vi "Transconductance state machine.vi"() -> ()   [LabVIEW 2016, in "Tranconductance SM.lvclass"]
uses:
  Tranconductance SM.lvclass
  <userlib>/LevyLab/Levylab Instruments/SMOs/Configuration/Configuration.lvclass
  <vilib>/Utility/sysdir.llb/System Directory Type.ctl
  Typedefs/Blob File--Cluster.ctl
  <userlib>/LevyLab/XY Utilities/Typedefs/Interpolation Configuration--cluster.ctl
  <userlib>/LevyLab/XY Utilities/subVIs/Remove Outliers (multiple).vi
  <userlib>/LevyLab/XY Utilities/subVIs/Zero Phase Lowpass Filter (multiple).vi
  <userlib>/LevyLab/XY Utilities/subVIs/Multiply float (multiple).vi
  <userlib>/LevyLab/XY Utilities/subVIs/Subtract float (multiple).vi
  <userlib>/LevyLab/XY Utilities/subVIs/Derivative (multiple).vi
  <userlib>/LevyLab/XY Utilities/subVIs/Interpolate (single).vi
  <vilib>/regexp/Match Regular Expression.xnode
  <vilib>/Analysis/NI_AAL_SigProc.lvlib
  <userlib>/LevyLab/Graph Utilities/graph_utilities.lvclass
  <userlib>/LevyLab/LV to ITX/Data.ITX/Data.ITX.lvclass
  <vilib>/Analysis/NI_AALPro.lvlib
  <userlib>/LevyLab/XY Utilities/xy_utilities.lvlib
  <userlib>/LevyLab/XY Utilities/subVIs/Shift Zero (single).vi
  <userlib>/LevyLab/LV to ITX/Data.TDMS/Data.TDMS.lvclass
  <userlib>/LevyLab/XY Utilities/subVIs/Resample (single).vi
  <userlib>/LevyLab/XY Utilities/subVIs/Subset (single).vi
panel:
  out "Current State":string
  in  "Clear Graphs & Stop":bool=TRUE
  in  "line cut":enum16{"Conductance", "Transconductance"}(ring)
  in  "Tab Control 2":T1(tab)
  out "Vertical Line Cut":cluster{"N1 (B field)":dbl[], dbl[]}[](graph)
  out "B field (T)":dbl=5.33284074074074
  out "vertical line cut \ncursor index":i32
  out "Horizontal Line Cut":cluster{"N1 (B field)":dbl[], dbl[]}[](graph)
  out "Vsg (V)":dbl=0.0006378350000000002 format="%#_6p"
  out "horizontal line cut\ncursor index":i32
  in  "Refresh":bool
  in  "Tab Control":T2(tab)
  in  "Load Notes":bool
  in  "B":u16(ring) items=["OFF", "Magnet Field", "Temperature", "Magnet", "Time", "Vsg", "X1", "Y1", "X2", "Y2", "X3", "Y3", "X4", "Y4", "X5", "Y5", "X6", "Y6", "X7", "Y7", "X8", "Y8"]
  in  "Vsg":u16(ring) items=["OFF", "Magnet Field", "Temperature", "Magnet", "Time", "Vsg", "X1", "Y1", "X2", "Y2", "X3", "Y3", "X4", "Y4", "X5", "Y5", "X6", "Y6", "X7", "Y7", "X8", "Y8"]
  in  "CURRENT":u16(ring) items=["OFF", "Magnet Field", "Temperature", "Magnet", "Time", "Vsg", "X1", "Y1", "X2", "Y2", "X3", "Y3", "X4", "Y4", "X5", "Y5", "X6", "Y6", "X7", "Y7", "X8", "Y8"]
  in  "V2":u16(ring) items=["OFF", "Magnet Field", "Temperature", "Magnet", "Time", "Vsg", "X1", "Y1", "X2", "Y2", "X3", "Y3", "X4", "Y4", "X5", "Y5", "X6", "Y6", "X7", "Y7", "X8", "Y8"]
  in  "Read TDMS Data":bool=TRUE
  in  "TDMS Path":path=path "G:/My Drive/ansom/Data/MNK/SA03018H.20170509/6 - sweep B, Vsg"
  in  "Load Wavenames":bool
  in  "V1":u16(ring) items=["OFF", "Magnet Field", "Temperature", "Magnet", "Time", "Vsg", "X1", "Y1", "X2", "Y2", "X3", "Y3", "X4", "Y4", "X5", "Y5", "X6", "Y6", "X7", "Y7", "X8", "Y8"]
  in  "Blob File Path":path=path "P:/users1/kirkendall/data/superlattice blob files/SA03018F.20171127_17B - sweep B, Vsg lockin, superlattice_original_6,8-4.blob"
  in  "Read Blob Data":bool
  in  "B field in T?":bool=TRUE
  in  "Indices":T3={"N1 (x axis)"=3, "N2"=19, "N3"=4, "N4"=5, "V1"=14, "V2"=4, "V3"=10, "V4"=13, "CURRENT"=6, "Vsg"=1}
  in  "ITX File or Folder Path":path=path "G:/My Drive/ansom/Data/MNK/SA03018H.20170509/6 - sweep B, Vsg"
  in  "File offset":i32
  in  "File length":i32=1000
  in  "single ended?":bool=TRUE
  in  "Read ITX Data":bool=TRUE
  out "Conductance vs Vsg":cluster{"N1 (B field)":dbl[], dbl[]}[](graph)
  out "Notes":string="IGOR\nX// Date: 2/8/2017 10:35 PM\nX// B=18T --> 0T, 0.05 T/min\nX// large axis: 157 -- 177, 10 deg steps\nX// small axis: 167\nX// sweep Vsg: 50mV to 170mV, 250uV steps\nX// Vbg=0.3V\nX// T<50mK\nX// \nX// lockin settings: \nX// tc=0.3s\nX// order=4\nX// prefilters OFF\nX// \nX// 0: 1, voltage\nX// 1: 2, current, 100uV AC 240uV DC, 13 Hz\nX// 2: 3, voltage\nX// 3: 4, voltage\nX// 4: 5, current\nX// 5: 7, voltage\nX//  \nX// KH gain=100x, shunt resistor=50kOhm\nX// \nX// axis1=157.013000\nX// axis2=166.999000\n\n\n\n\n\n\n\n\n\n\n\n\n\n\n\n\n\n\n\n\n\n\n\n\n\n\n\n\n\n\n\n\n\n\n\n\n\n\n\n\n\n\nX \nX Display/R 'time.SA02836H.20170110.000242'\nX AppendToGraph 'Vsg.SA02836H.20170110.000242'\nX AppendToGraph 'T.SA02836H.20170110.000242'\nX AppendToGraph 'B.SA02836H.20170110.000242'\nX AppendToGraph 'X0.SA02836H.20170110.000242'\nX AppendToGraph 'Y0.SA02836H.20170110.000242'\nX AppendToGraph 'X1.SA02836H.20170110.000242'\nX AppendToGraph 'Y1.SA02836H.20170110.000242'\nX AppendToGraph 'X2.SA02836H.20170110.000242'\nX AppendToGraph 'Y2.SA02836H.20170110.000242'\nX AppendToGraph 'X3.SA02836H.20170110.000242'\nX AppendToGraph 'Y3.SA02836H.20170110.000242'\nX AppendToGraph 'X4.SA02836H.20170110.000242'\nX AppendToGraph 'Y4.SA02836H.20170110.000242'\nX AppendToGraph 'X5.SA02836H.20170110.000242'\nX AppendToGraph 'Y5.SA02836H.20170110.000242'\nX AppendToGraph 'B_rate.SA02836H.20170110.000242'\nX AppendToGraph 'R4t(e2/h).SA02836H.20170110.000242'\nX AppendToGraph 'axis1.SA02836H.20170110.000242'\nX AppendToGraph 'axis2.SA02836H.20170110.000242'\nX Label bottom \"x label\"\nX Label left \"y label\"\nX ModifyGraph rgb('time.SA02836H.20170110.000242')=(65280,0,0)\nX ModifyGraph rgb('Vsg.SA02836H.20170110.000242')=(65280,18432,0)\nX ModifyGraph rgb('T.SA02836H.20170110.000242')=(65280,35328,0)\nX ModifyGraph rgb('B.SA02836H.20170110.000242')=(65280,52224,0)\nX ModifyGraph rgb('X0.SA02836H.20170110.000242')=(60416,65280,0)\nX ModifyGraph rgb('Y0.SA02836H.20170110.000242')=(41984,65280,0)\nX ModifyGraph rgb('X1.SA02836H.20170110.000242')=(25088,65280,0)\nX ModifyGraph rgb('Y1.SA02836H.20170110.000242')=(8192,65280,0)\nX ModifyGraph rgb('X2.SA02836H.20170110.000242')=(0,65280,10240)\nX ModifyGraph rgb('Y2.SA02836H.20170110.000242')=(0,65280,28672)\nX ModifyGraph rgb('X3.SA02836H.20170110.000242')=(0,65280,45568)\nX ModifyGraph rgb('Y3.SA02836H.20170110.000242')=(0,65280,62464)\nX ModifyGraph rgb('X4.SA02836H.20170110.000242')=(0,50176,65280)\nX ModifyGraph rgb('Y4.SA02836H.20170110.000242')=(0,31744,65280)\nX ModifyGraph rgb('X5.SA02836H.20170110.000242')=(0,14848,65280)\nX ModifyGraph rgb('Y5.SA02836H.20170110.000242')=(2048,0,65280)\nX ModifyGraph rgb('B_rate.SA02836H.20170110.000242')=(20480,0,65280)\nX ModifyGraph rgb('R4t(e2/h).SA02836H.20170110.000242')=(38912,0,65280)\nX ModifyGraph rgb('axis1.SA02836H.20170110.000242')=(55808,0,65280)\nX ModifyGraph rgb('axis2.SA02836H.20170110.000242')=(65280,0,58368)\nX Legend/C/N=text0/J \"\\\\s('time.SA02836H.20170110.000242') time\\r\\\\s('Vsg.SA02836H.20170110.000242') Vsg\\r\\\\s('T.SA02836H.20170110.000242') T\\r\\\\s('B.SA02836H.20170110.000242') B\\r\\\\s('X0.SA02836H.20170110.000242') X0\\r\\\\s('Y0.SA02836H.20170110.000242') Y0\\r\\\\s('X1.SA02836H.20170110.000242') X1\\r\\\\s('Y1.SA02836H.20170110.000242') Y1\\r\\\\s('X2.SA02836H.20170110.000242') X2\\r\\\\s('Y2.SA02836H.20170110.000242') Y2\\r\\\\s('X3.SA02836H.20170110.000242') X3\\r\\\\s('Y3.SA02836H.20170110.000242') Y3\\r\\\\s('X4.SA02836H.20170110.000242') X4\\r\\\\s('Y4.SA02836H.20170110.000242') Y4\\r\\\\s('X5.SA02836H.20170110.000242') X5\\r\\\\s('Y5.SA02836H.20170110.000242') Y5\\r\\\\s('B_rate.SA02836H.20170110.000242') B_rate\\r\\\\s('R4t(e2/h).SA02836H.20170110.000242') R4t (e2/h)\\r\\\\s('axis1.SA02836H.20170110.000242') axis 1\\r\\\\s('axis2.SA02836H.20170110.000242') axis 2\"\nX ModifyGraph mirror(bottom)=1\nX ModifyGraph width=216\nX ModifyGraph height={Aspect,0.6}\nX ModifyGraph Log(bottom)=0\nX ModifyGraph Log(left)=0\nX \n"
  out "B Field Array":dbl[](array[numeric])
  in  "Resample":bool
  in  "mu offset":dbl
  in  "Multiply":bool
  in  "alpha":dbl=1.0 format="%#_13g"
  in  "Derivative Type":enum16{"dy/dx vs x", "dx/dy vs y"}(ring)
  in  "Interval Units":enum16{"Points", "Data"}(ring)
  in  "Interval":dbl=2.0
  in  "Lower":dbl
  in  "Upper":dbl
  in  "Filter?":bool=TRUE
  in  "restrict range?":bool
  in  "flatten trans?":bool
  in  "cutoff period":dbl
  out "Cond intensity":dbl[][](graph)
  out "Conductance":cluster{"N1 (B field)":dbl[], dbl[]}[](graph)
  in  "Decimation":i32=1
  in  "start B":dbl=-18.0
  in  "end B":dbl
  in  "offset cond (horizontal)":dbl=-0.001
  in  "Offset":i32
  out "Transconductance":T4(graph)
  out "Transcond Intensity":dbl[][](graph)
  in  "offset trans (vertical)":dbl
  out "modified trans":cluster{"N1 (B field)":dbl[], dbl[]}[](graph)
  in  "threshold":dbl=2.0 format="%0.2f"
  in  "width":i32=40 min=3
  in  "X Low":dbl format="%#_6p"
  in  "X High":dbl=0.0015 format="%#_6p"
  out "Flattened Trans":dbl[][](graph)
  in  "manual offset array":dbl[](array[numeric])
  out "number of curves":i32=535
  in  "add manual offset?":T5(ring)=enum."No manual offset"
  in  "mirror?":bool
  in  "flip mirror":bool
  in  "offset":dbl=-18.0
  in  "write blob?":bool
  in  ".blob file \nconductance":enum16{"original cond", "modified cond"}(ring)
  in  "blob note":string
  in  "cond int X,Y,Z Scale Names":string[](array[string])=["\\f02B \\f00(T)", "\\f02V\\f00\\Bsg\\M (mV)", "\\f02G \\f00 (e\\S2\\M/h)"]
  in  "trans cond X,Y,Z Scale Names":string[](array[string])=["\\f02B \\f00(T)", "\\f02V\\f00\\Bsg\\M (mV)", "\\f02dG/dV\\f00\\Bsg\\M (arb. units)"]
  in  "export to igor path":path=path "C:/Users/ansom/OneDrive/Manuscripts.ansom/1D superlattice/Helical figures/data/igor files"
  in  "intensity input ITX commands":string="Display;AppendImage '#wave2D#'\nModifyGraph width=144,height={Aspect,1}\nLabel bottom \"#labelX#\"\nLabel left \"#labelY#\"\nModifyGraph mirror=1\nModifyGraph prescaleExp(left)=3\nColorScale/C/N=text0/F=0/H=5/A=MC image='#wave2D#'\nColorScale/C/N=text0 \"#labelZ#\"\nModifyGraph margin(right)=108\nColorScale/C/N=text0/X=80.00/Y=-30.00 heightPct=50\nColorScale/C/N=text0/D=0.5\nModifyGraph axThick(left)=0.5\nColorScale/C/N=text0 tickThick=0.50\nColorScale/C/N=text0 frame=0.50\nModifyGraph axThick=0.5"
  in  "Enum":T6(ring)=enum."Flattened trans intensity"
  in  "xy graph X,Y,Z Scale Names":string[](array[string])=["\\f02V\\f00\\Bsg\\M (mV)", "\\f02G \\f00 (e\\S2\\M/h)", ""]
  in  "xy graph data":T7(ring)=enum."trans all"
  in  "xy input ITX commands":string="Display 'y_#wave#' vs 'x_#wave#'\nAppendToGraph 'y_#wave#' vs 'x_#wave#'\nLabel bottom \"#labelX#\"\nLabel left \"#labelY#\"\nModifyGraph rgb=(0,15872,65280)\n\\\\s('y_#wave#') #label#\nModifyGraph mirror=1\nModifyGraph width={Aspect,1.5}\nModifyGraph height=144\nModifyGraph Log(bottom)=#bottomlog#\nModifyGraph Log(left)=#leftlog#\nModifyGraph lsize=0.5\nLegend/K/N=text0\nModifyGraph axThick(left)=0.5\nModifyGraph axThick=0.5\nTextBox/C/N=text0/X=80.00/Y=5.00\nTextBox/C/N=text1/X=5.00/Y=5.00\nModifyGraph grid(left)=1\nModifyGraph prescaleExp(bottom)=3"
  in  "Export igor files":bool
  in  "Stop":bool
  # "Conductance curve, select using cursor on transconductance or conductance intensity plot"
  # "Data"
  # "Configure Read TDMS File"
  # "Configure Read Blob File"
  # "Configure Read ITX File"
  # "creates conductance plot\ny axis: current/(V1-V2)\nx axis: Vsg"
  # "choose N1 to be the B field, or other slow parameter\nfor intensity plots"
  # "Modify Conductance data"
  # "Transconductance Derivative Parameters"
  # "Resample"
  # "Before hitting resample choose zero point in the \nhorizontal line cut graph"
  # "To apply changes press the 'Refresh' button"
  # "Peak finding"
  # "Interpolating"
  # "Mirror"
  # "italic variable (normal unit)\n\\f02 X\\Bsub\\M\\f00 (unit\\S2\\M)"
  # "\\f02dG/dV\\f00\\Bsg\\M (arb. units)"
  # "dG/dmu\n\\f02 dG/d\\F'Arial Greek'ì \\f00(S/eV)"
  # "mu\n\\f02\\F'Arial Greek'ì \\f00 (meV)"
  # "\\f02B \\f00(T)"
  # "\\f02V\\f00\\Bsg\\M (meV)"
  # "\\f02G \\f00(e\\S2\\M/h)"
  # "make rainbow traces:\nModifyGraph rgb('y_#wave#')=(#r#,#g#,#b#)"
  # "Display 'y_#wave#' vs 'x_#wave#'\nAppendToGraph 'y_#wave#' vs 'x_#wave#'\nLabel bottom \"#labelX#\"\nLabel left \"#labelY#\"\nModifyGraph rgb('y_#wave#')=(#r#,#g#,#b#)\n\\\\s('y_#wave#') #label#\nModifyGraph mirror=1\nModifyGraph width=216\nModifyGraph height={Aspect,0.6}\nModifyGraph Log(bottom)=#bottomlog#\nModifyGraph Log(left)=#leftlog#"
  # "Display;AppendImage '#wave2D#'\nModifyGraph width=144,height={Aspect,1}\nLabel bottom \"#labelX#\"\nLabel left \"#labelY#\"\nModifyGraph mirror=1\nModifyGraph prescaleExp(left)=3\nColorScale/C/N=text0/F=0/H=5/A=MC image='#wave2D#'\nColorScale/C/N=text0 \"#labelZ#\"\nModifyGraph margin(right)=108\nColorScale/C/N=text0/X=80.00/Y=-30.00 heightPct=50"
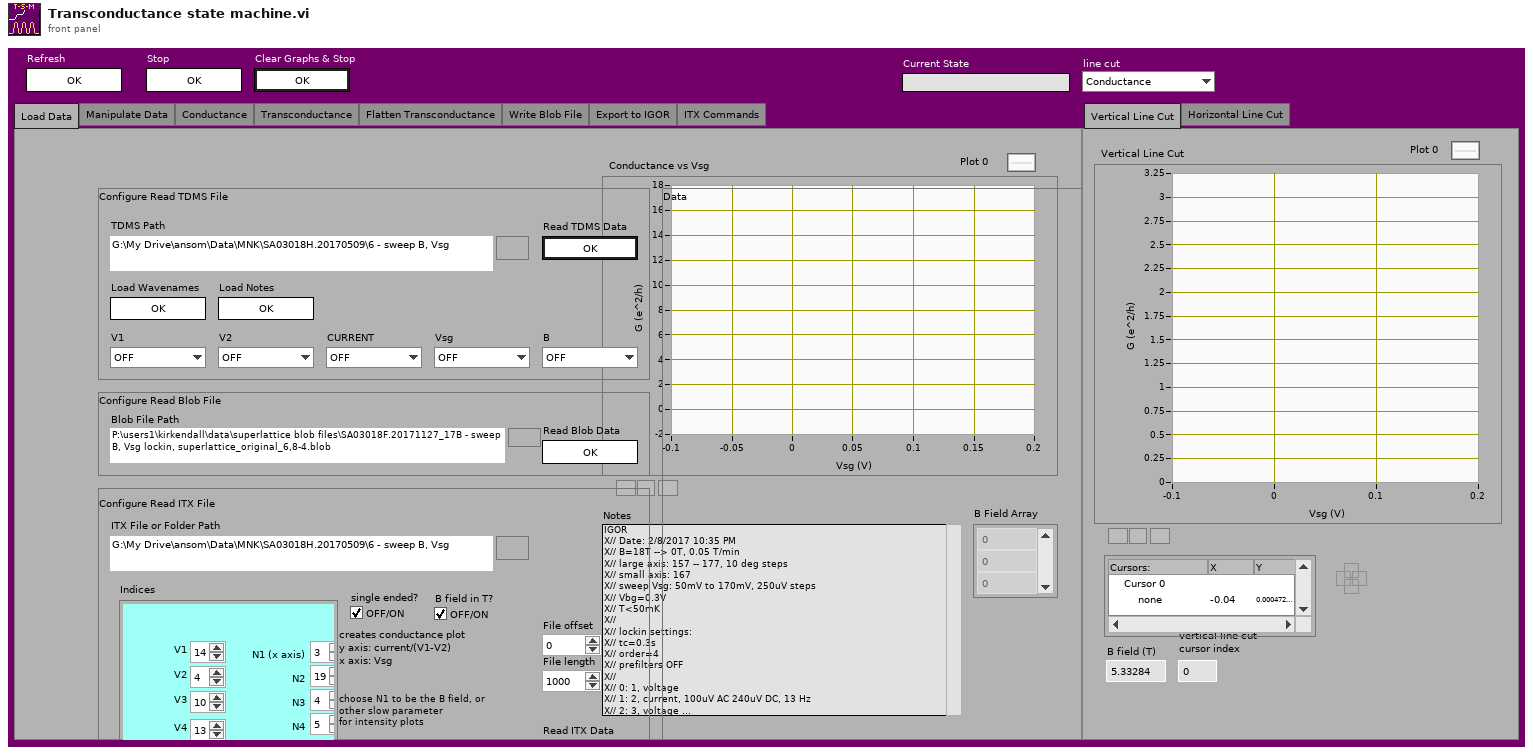
[diagram p1: front panel]
types:
  T1 = enum32{"Vertical Line Cut", "Horizontal Line Cut"}
  T2 = enum32{"Load Data", "Manipulate Data", "Conductance", "Transconductance", "Flatten Transconductance", "Write Blob File", "Export to IGOR", "ITX Commands"}
  T3 = cluster{"N1 (x axis)":i32, "N2":i32, "N3":i32, "N4":i32, "V1":i32, "V2":i32, "V3":i32, "V4":i32, "CURRENT":i32, "Vsg":i32}
  T4 = cluster{"Vfast":dbl[], "Decimated Array":dbl[]}[]
  T5 = enum16{"Only manual offset", "Add manual offset", "No manual offset"}
  T6 = enum16{"Cond intensity", "xy", "Trans intensity", "Flattened trans intensity"}
  T7 = enum16{"cond all", "trans all", "vert cut", "horz cut"}
  T8 = enum32{"vertical line cut", "Horizontal line cut"}
  T9 = enum32{"invalid app kind", "Development System", "Run Time System", "Student Edition", "Embedded LabVIEW", "Evaluation", "Custom"}
  T10 = enum32{"Invalid", "Standard", "Closed", "Hidden", "Minimized", "Maximized"}
  T11 = typedef "Tranconductance SM.lvclass/Blob File--Cluster.ctl" = cluster{"Vsg offset and mult":cluster{dbl, dbl}, "number of curves":i32, "A vs D":cluster{dbl[], dbl[]}[], "N1 (B field)":dbl[], "B offset and mult":cluster{"N1":dbl, dbl}, "Comments":string}
  T12 = typedef "xy_utilities.lvlib/Interpolation Configuration--cluster.ctl" = cluster{"X Low":dbl, "X High":dbl, "X Step":dbl, "Fake Point":dbl}
  T13 = cluster{"2D Array":dbl[][], "X 1D Array":dbl[], "Y 1D Array":dbl[]}
  T14 = cluster{"Core":cluster{"Current VI Reference":refnum<vi>, "Close Panel on Exit?":bool}, "Original Conductance":cluster{"Vfast":dbl[], "Decimated Array":dbl[]}[], "Modified Conductance":cluster{"Vfast":dbl[], "Decimated Array":dbl[]}[], "Transconductance":cluster{"Vfast":dbl[], "Decimated Array":dbl[]}[], "Modified Transconductance":cluster{"Vfast":dbl[], "Decimated Array":dbl[]}[], "Cond Intensity":dbl[][], "Transcond Intensity":dbl[][], "N Array":cluster{"N1":dbl, "N2":dbl, "N3":dbl, "N4":dbl}[], "N1 (B field)":dbl[], "Vsg offset and mult":cluster{dbl, dbl}, "B offset and mult":cluster{dbl, dbl}, "number of curves":i32, "cursor plot":i32, "cursor index":i32, "resample index":i32, "Configuration":refnum<class "Configuration.lvclass">, "Config Cluster":cluster{"ITX File or Folder Path":path, "Blob File Path":path}, "TDMS Path":path}
  T15 = cluster{"ITX File or Folder Path":path, "Blob File Path":path}
  T16 = cluster{"N1":dbl, "N2":dbl, "N3":dbl, "N4":dbl}[]
  T17 = cluster{"Current VI Reference":refnum<vi>, "Close Panel on Exit?":bool}
  T18 = typedef "System Directory Type.ctl" = i32
  T19 = typedef "LVOffsetAndMultiplierTypeDef.ctl" = cluster{"Offset":dbl, "Multiplier":dbl}
  T20 = enum16{"open", "replace", "create", "open or create", "replace or create", "replace or create with confirmation"}
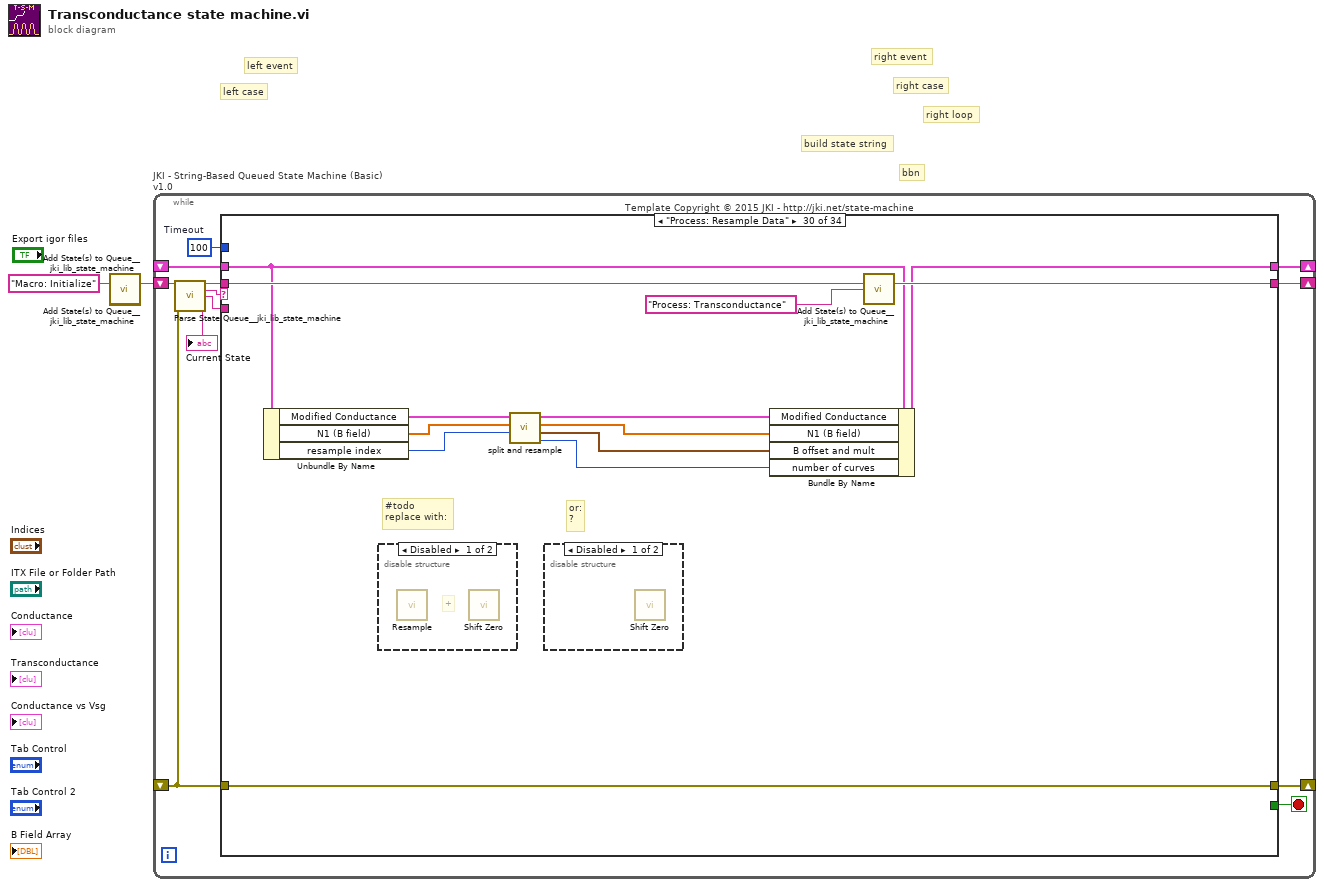
[diagram p0: block diagram]
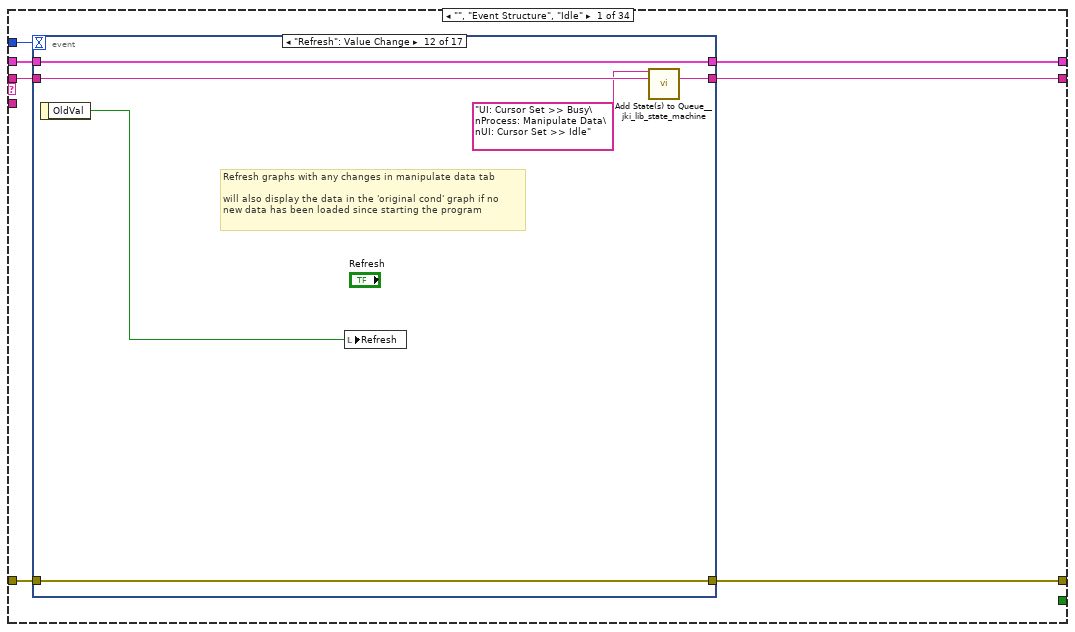
[diagram p2: hidden frame]
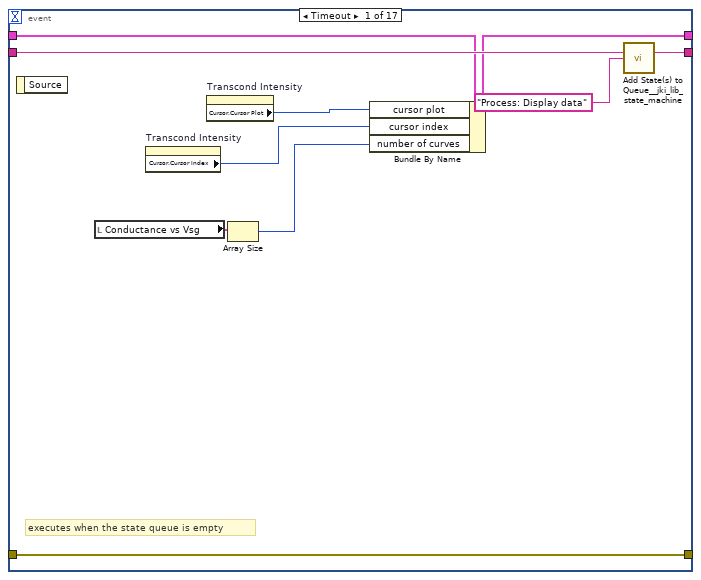
[diagram p3: hidden frame]
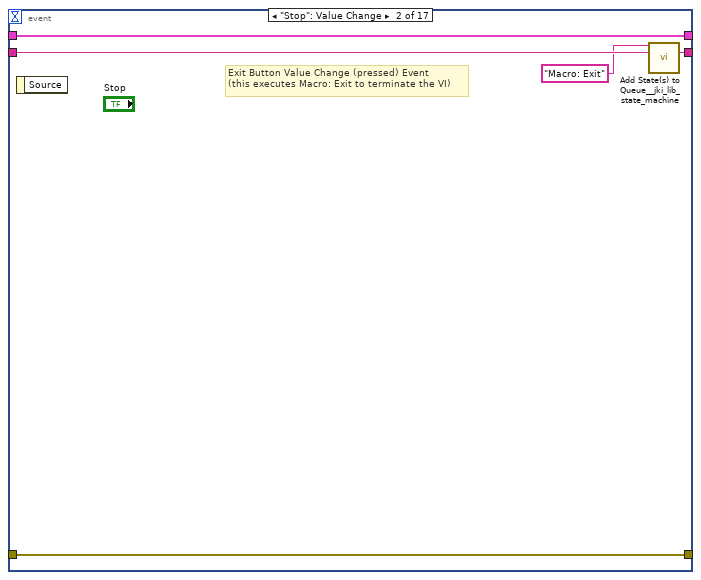
[diagram p4: hidden frame]
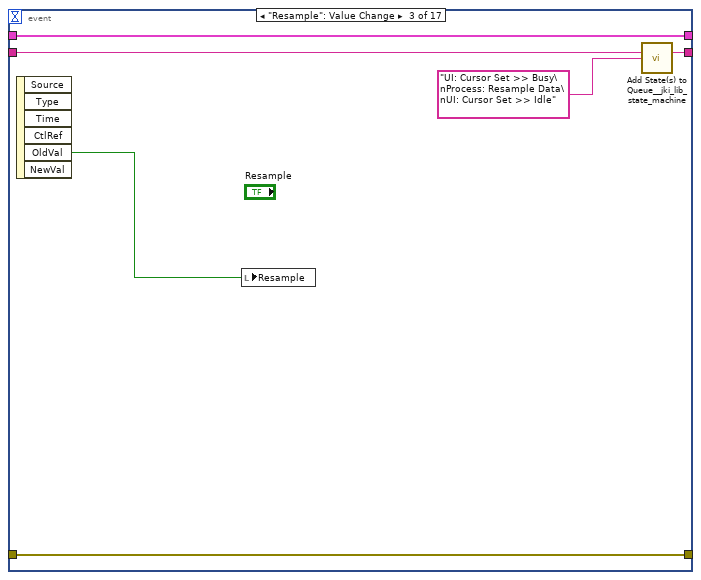
[diagram p5: hidden frame]
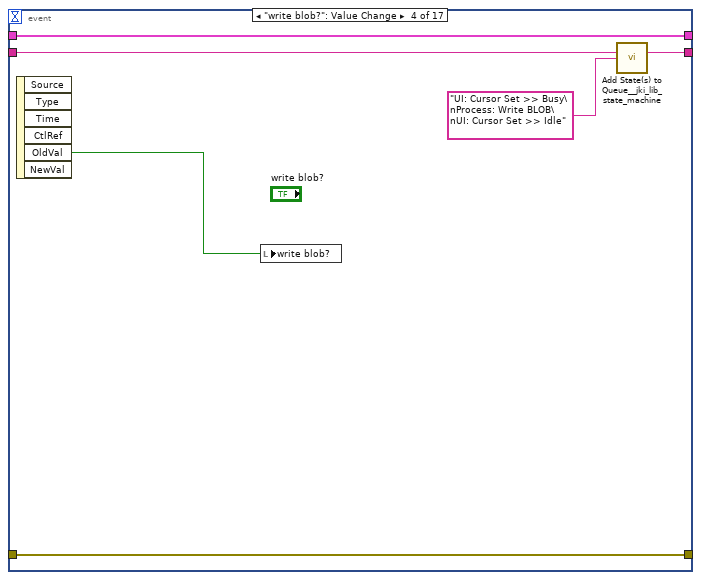
[diagram p6: hidden frame]
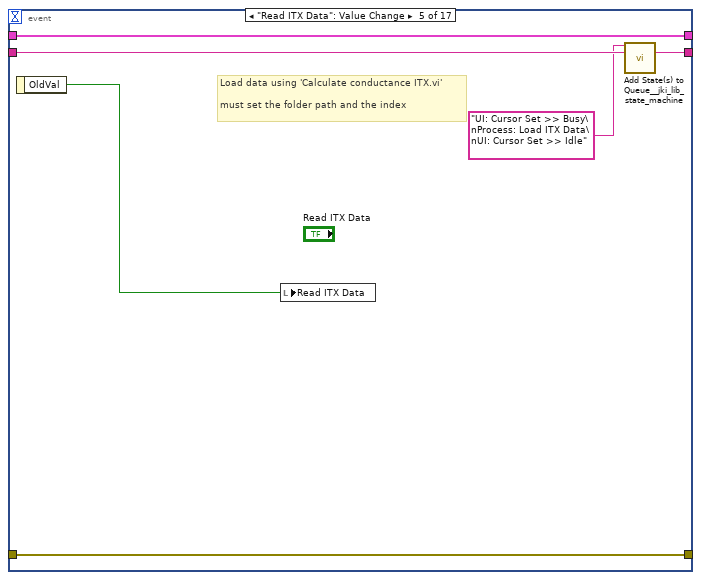
[diagram p7: hidden frame]
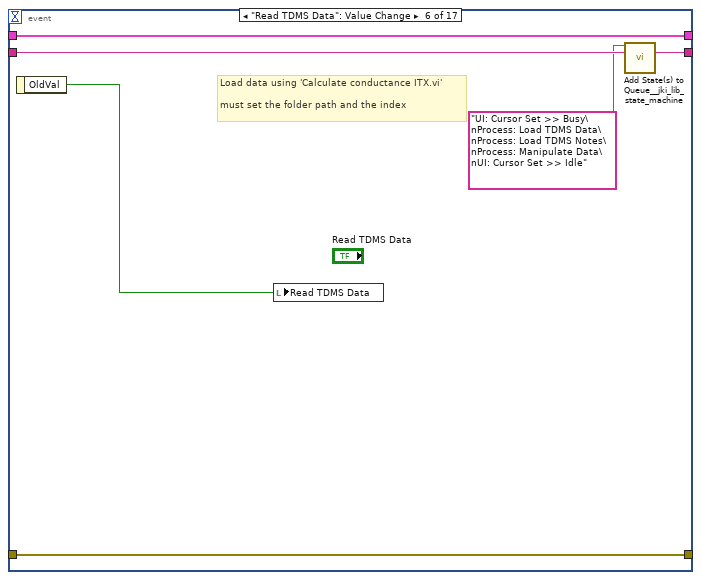
[diagram p8: hidden frame]
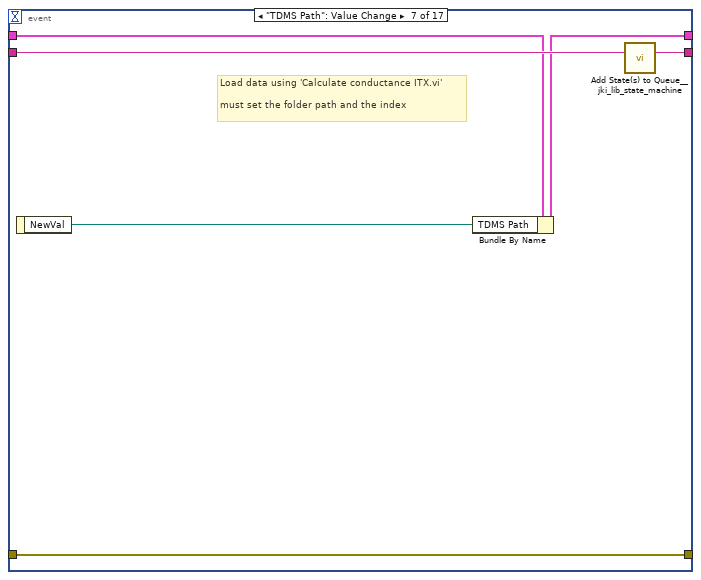
[diagram p9: hidden frame]
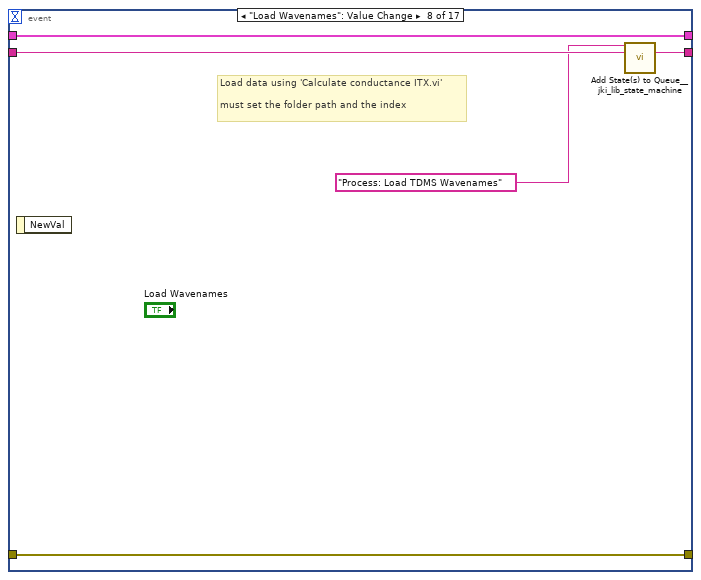
[diagram p10: hidden frame]
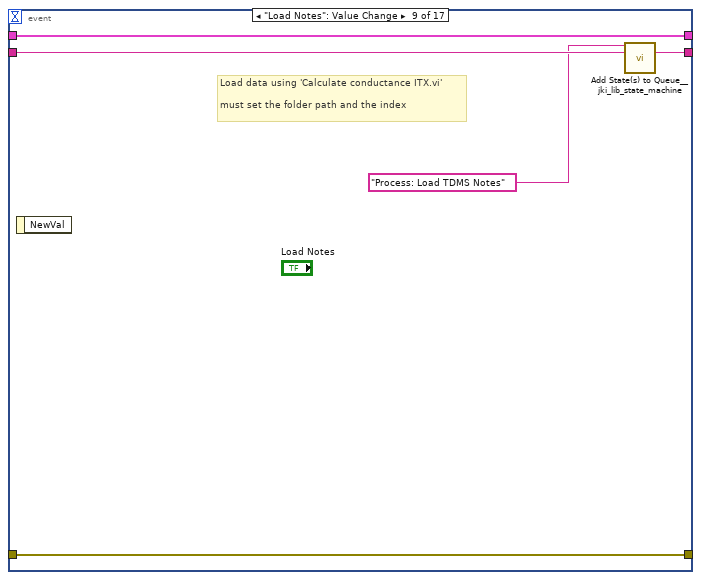
[diagram p11: hidden frame]
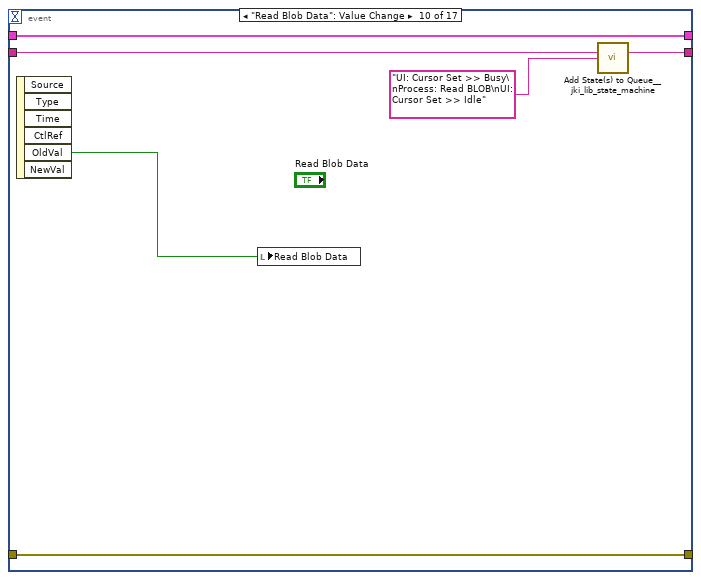
[diagram p12: hidden frame]
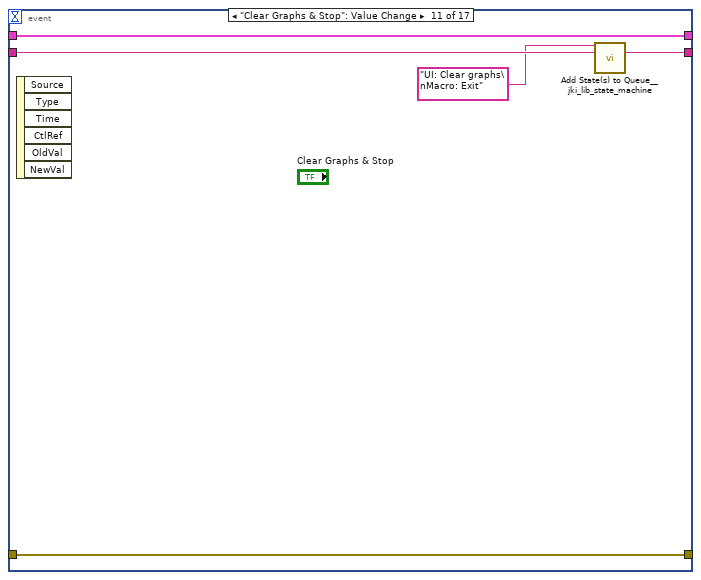
[diagram p13: hidden frame]
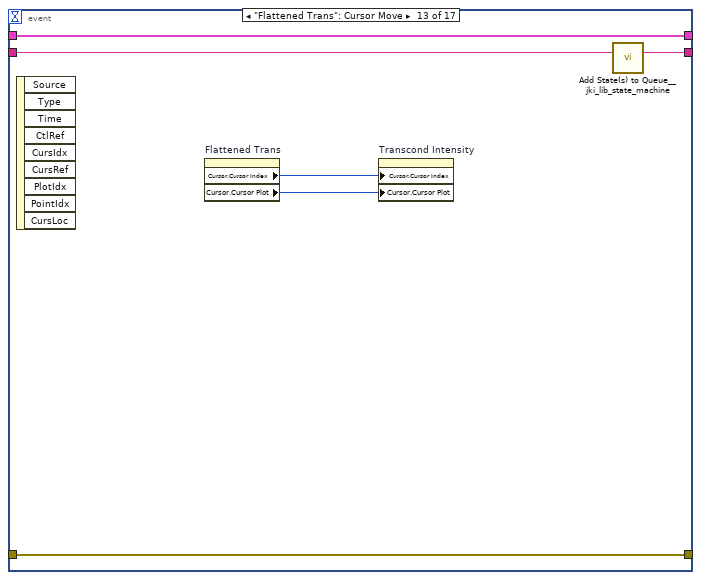
[diagram p14: hidden frame]
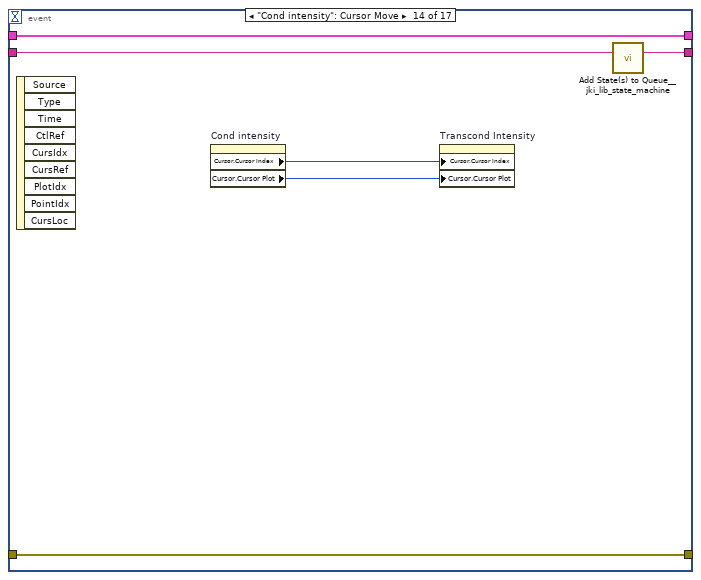
[diagram p15: hidden frame]
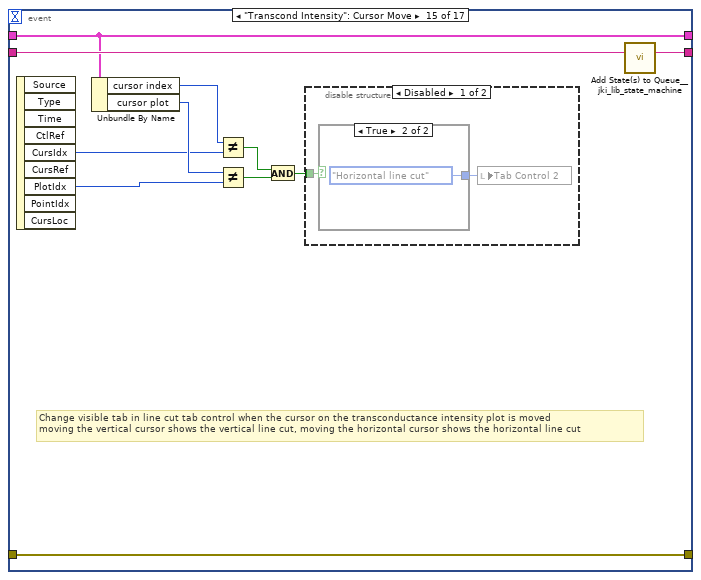
[diagram p16: hidden frame]
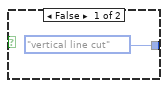
[diagram p17: hidden frame]
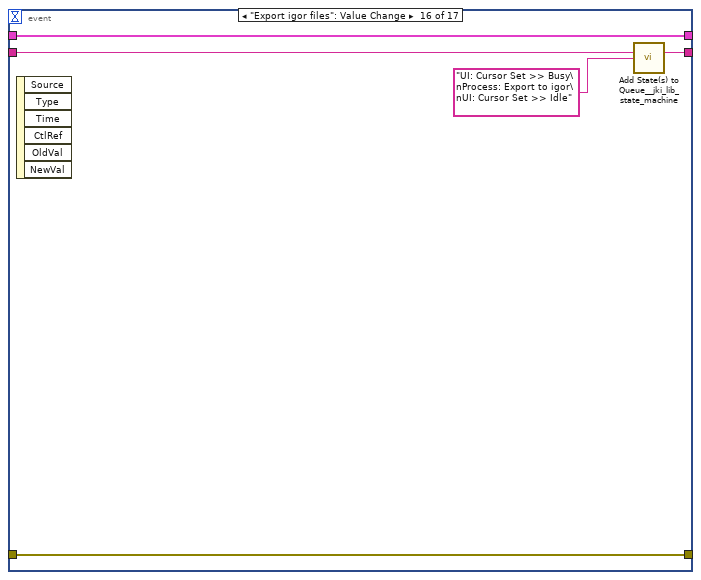
[diagram p19: hidden frame]
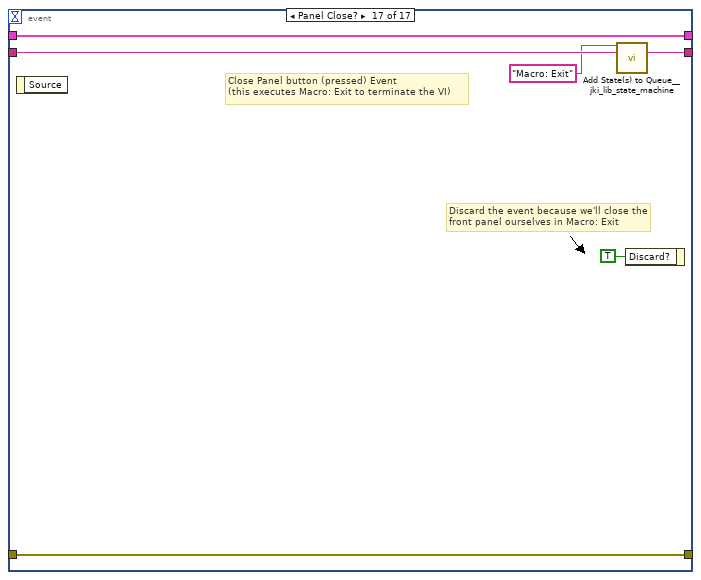
[diagram p20: hidden frame]
diagram:
  # "bbn"
  # "build state string"
  # "right loop"
  # "right case"
  # "right event"
  # "left event"
  # "left case"
  n1 = call <vilib>:"Add State(s) to Queue__jki_lib_state_machine.vi"("State(s) in (\"\")"="Macro: Initialize") -> ("States Out"=w2:string)  [unwired: 14 in]
  n2 = call <vilib>:"Add State(s) to Queue__jki_lib_state_machine.vi"() -> ()  [unwired: 15 in, 1 out]
  n3 = while "JKI - String-Based Queued State Machine (Basic) v1.0" {
    shift-right: [w6] -> _
    shift-left: _ -> [w5]
    shift-right: [w9] -> _
    shift-left: _ -> [w3]
    shift-right: [w8] -> _
    shift-left: w2 -> [w10]
    stop <- w7 stop-if-true
    w4 = 100  # Timeout
    # "Template Copyright © 2015 JKI - http://jki.net/state-machine"
    n4 = call <vilib>:"Parse State Queue__jki_lib_state_machine.vi"("State Queue"=w10, "Error In (no error)"=w3) -> ("Remaining States"=w12:string, "Current State"=w13:string, "Arguments"=w11:string)  [unwired: 11 in]
    "Current State" <- w13
    n5 = case shown="\"Process: Resample Data\"" w13 {
      selector: w13 -> [_ _ w135 _ _ _ _ _ _ _ _ _ _ _ _ _ _ _ _ _ _ _ _ _ _ _ _ _ _ _ _ _ _ _]
      tunnel: w12 -> [w20 w134 w139 w157 w163 w168 w172 w194 w206 w220 w232 w238 w242 w260 w273 w281 w292 w316 w322 w327 w338 w342 w385 w427 w476 w483 w538 w559 w578 w616 w628 w639 w721 w783]
      tunnel: w11 -> [_ _ _ _ _ _ _ _ _ _ _ _ _ _ _ w276 w286 _ _ _ _ _ _ _ _ _ _ _ _ _ _ _ _ _]
      tunnel: w5 -> [w18 w131 w137 w148 w160 w166 w169 _ w204 w216 w230 w233 w239 w258 w270 w279 w288 w317 w319 w324 w335 w339 w366 w409 w472 w477 w513 w553 w569 w612 w617 w636 w682 w784]
      tunnel: [w17 w132 w141 w154 errorcluster {"status"=FALSE, "code"=0, "source"=""} ("error out") w165 w170 w192 w199 w211 w225 w234 w240 w250 w271 w277 w289 w318 w320 w325 w336 w340 w351 w404 w470 w480 w526 w545 w570 w613 w621 w637 w711 w781] -> w9
      tunnel: w3 -> [w14 w132 w140 w154 w159 w165 w170 w192 w200 w214 w226 w235 w240 w251 w271 w278 w290 w318 w320 w325 w336 w340 w351 w405 w471 w478 w527 w546 w564 w613 w622 w637 w711 w781]
      tunnel: [w19 w133 w138 w156 w162 w167 w171 w193 w205 w219 w231 w237 w241 w259 w272 w280 w291 w315 w321 w326 w337 w341 w384 w426 w475 w482 w537 w558 w577 w615 w627 w638 w720 w782] -> w8
      tunnel: [_ _ _ _ _ TRUE _ _ _ _ _ _ _ _ _ _ _ _ _ _ _ _ _ _ _ _ _ _ _ _ _ _ _ _] -> w7
      tunnel: [w16 w131 w137 w155 w160 w166 w169 w179 w203 w215 w229 w233 w239 w256 w270 w279 w288 w317 w319 w324 w335 w339 w382 w408 w472 w477 w513 w552 w574 w611 w626 w635 w704 w784] -> w6
      tunnel: w4 -> [w15 _ _ _ _ _ _ _ _ _ _ _ _ _ _ _ _ _ _ _ _ _ _ _ _ _ _ _ _ _ _ _ _ _]
      frame "", "Event Structure", "Idle" {
        n6 = event shown="[11] \"Refresh\": Value Change" {
          selector: _ -> [_ _ _ _ _ _ _ _ _ _ _ _ _ _ _ _ _]
          dyn-events: _ -> [_ _ _ _ _ _ _ _ _ _ _ _ _ _ _ _ _]
          timeout: w15 -> [_ _ _ _ _ _ _ _ _ _ _ _ _ _ _ _ _]
          tunnel: w20 -> [w30 w35 w39 w45 w53 w59 w65 w70 w75 w80 w85 w92 w93 w103 w115 w122 w130]
          tunnel: [w29 w34 w37 w44 w52 w58 w64 w69 w74 w79 w84 w91 w94 w102 w114 w121 w129] -> w19
          tunnel: w18 -> [w26 w32 w41 w47 w50 w56 w62 w67 w72 w81 w86 w89 w96 w104 w113 w124 w127]
          tunnel: [w28 w33 w40 w46 w51 w57 w63 w68 w73 w77 w82 w90 w95 w101 w108 w123 w128] -> w17
          tunnel: w14 -> [w28 w33 w40 w46 w51 w57 w63 w68 w73 w77 w82 w90 w95 w101 w108 w123 w128]
          tunnel: [w25 w32 w41 w47 w50 w56 w61 w67 w72 w81 w86 w89 w96 w104 w113 w124 w127] -> w16
          event Timeout {
            # "executes when the state queue is empty"
            n7 = event-data() -> ()  [unwired: 1 in, 1 out]
            n8 = local read "Conductance vs Vsg"() -> (w22:cluster{"N1 (B field)":dbl[], dbl[]}[])
            n9 = property on="Transcond Intensity" class="IntGraph (strict)"() -> ("Cursor.Cursor Index"=w23:i32)  [unwired: 2 in, 2 out]
            n10 = property on="Transcond Intensity" class="IntGraph (strict)"() -> ("Cursor.Cursor Plot"=w24:i32)  [unwired: 2 in, 2 out]
            n11 = Array Size(array=w22) -> (size(s)=w21:i32)
            n12 = Bundle By Name(cluster=w26, "cursor plot"=w24, "cursor index"=w23, "number of curves"=w21) -> (w25:T14)
            n13 = call <vilib>:"Add State(s) to Queue__jki_lib_state_machine.vi"("State(s) in (\"\")"=w30, "State(s) at Back (\"\")"="Process: Display data" ("State(s) at Back (\"\")")) -> ("States Out"=w29:string)  [unwired: 13 in]
          }
          event "Stop": Value Change {
            # "Exit Button Value Change (pressed) Event\n(this executes Macro: Exit to terminate the VI)"
            n14 = event-data() -> ()  [unwired: 1 in, 1 out]
            n15 = call <vilib>:"Add State(s) to Queue__jki_lib_state_machine.vi"("State(s) in Front (\"\")"="Macro: Exit", "State(s) in (\"\")"=w35) -> ("States Out"=w34:string)  [unwired: 13 in]
          }
          event "Resample": Value Change {
            n16 = event-data() -> ("OldVal"=w36:bool)  [unwired: 1 in, 5 out]
            n17 = local write "Resample"(w36) -> ()
            n18 = call <vilib>:"Add State(s) to Queue__jki_lib_state_machine.vi"("State(s) in (\"\")"=w39, "State(s) at Back (\"\")"="UI: Cursor Set >> Busy\nProcess: Resample Data\nUI: Cursor Set >> Idle" ("State(s) at Back (\"\")")) -> ("States Out"=w37:string)  [unwired: 13 in]
          }
          event "write blob?": Value Change {
            n19 = event-data() -> ("OldVal"=w42:bool)  [unwired: 1 in, 5 out]
            n20 = local write "write blob?"(w42) -> ()
            n21 = call <vilib>:"Add State(s) to Queue__jki_lib_state_machine.vi"("State(s) in (\"\")"=w45, "State(s) at Back (\"\")"="UI: Cursor Set >> Busy\nProcess: Write BLOB\nUI: Cursor Set >> Idle" ("State(s) at Back (\"\")")) -> ("States Out"=w44:string)  [unwired: 13 in]
          }
          event "Read ITX Data": Value Change {
            # "Load data using 'Calculate conductance ITX.vi'\n\nmust set the folder path and the index"
            n22 = event-data() -> ("OldVal"=w48:bool)  [unwired: 1 in]
            n23 = local write "Read ITX Data"(w48) -> ()
            n24 = call <vilib>:"Add State(s) to Queue__jki_lib_state_machine.vi"("State(s) in Front (\"\")"="UI: Cursor Set >> Busy\nProcess: Load ITX Data\nUI: Cursor Set >> Idle", "State(s) in (\"\")"=w53) -> ("States Out"=w52:string)  [unwired: 13 in]
          }
          event "Read TDMS Data": Value Change {
            # "Load data using 'Calculate conductance ITX.vi'\n\nmust set the folder path and the index"
            n25 = event-data() -> ("OldVal"=w54:bool)  [unwired: 1 in]
            n26 = local write "Read TDMS Data"(w54) -> ()
            n27 = call <vilib>:"Add State(s) to Queue__jki_lib_state_machine.vi"("State(s) in Front (\"\")"="UI: Cursor Set >> Busy\nProcess: Load TDMS Data\nProcess: Load TDMS Notes\nProcess: Manipulate Data\nUI: Cursor Set >> Idle", "State(s) in (\"\")"=w59) -> ("States Out"=w58:string)  [unwired: 13 in]
          }
          event "TDMS Path": Value Change {
            # "Load data using 'Calculate conductance ITX.vi'\n\nmust set the folder path and the index"
            n28 = event-data() -> ("NewVal"=w60:path)  [unwired: 1 in]
            n29 = Bundle By Name(cluster=w62, "TDMS Path"=w60) -> (w61:T14)
            n30 = call <vilib>:"Add State(s) to Queue__jki_lib_state_machine.vi"("State(s) in (\"\")"=w65) -> ("States Out"=w64:string)  [unwired: 14 in]
          }
          event "Load Wavenames": Value Change {
            # "Load data using 'Calculate conductance ITX.vi'\n\nmust set the folder path and the index"
            n31 = event-data() -> ()  [unwired: 1 in, 1 out]
            n32 = call <vilib>:"Add State(s) to Queue__jki_lib_state_machine.vi"("State(s) in Front (\"\")"="Process: Load TDMS Wavenames" ("State(s) in Front (\"\")"), "State(s) in (\"\")"=w70) -> ("States Out"=w69:string)  [unwired: 13 in]
          }
          event "Load Notes": Value Change {
            # "Load data using 'Calculate conductance ITX.vi'\n\nmust set the folder path and the index"
            n33 = event-data() -> ()  [unwired: 1 in, 1 out]
            n34 = call <vilib>:"Add State(s) to Queue__jki_lib_state_machine.vi"("State(s) in Front (\"\")"="Process: Load TDMS Notes" ("State(s) in Front (\"\")"), "State(s) in (\"\")"=w75) -> ("States Out"=w74:string)  [unwired: 13 in]
          }
          event "Read Blob Data": Value Change {
            n35 = event-data() -> ("OldVal"=w76:bool)  [unwired: 1 in, 5 out]
            n36 = local write "Read Blob Data"(w76) -> ()
            n37 = call <vilib>:"Add State(s) to Queue__jki_lib_state_machine.vi"("State(s) in (\"\")"=w80, "State(s) at Back (\"\")"="UI: Cursor Set >> Busy\nProcess: Read BLOB\nUI: Cursor Set >> Idle" ("State(s) at Back (\"\")")) -> ("States Out"=w79:string)  [unwired: 13 in]
          }
          event "Clear Graphs & Stop": Value Change {
            n38 = event-data() -> ()  [unwired: 1 in, 6 out]
            n39 = call <vilib>:"Add State(s) to Queue__jki_lib_state_machine.vi"("State(s) in Front (\"\")"="UI: Clear graphs\nMacro: Exit" ("State(s) in Front (\"\")"), "State(s) in (\"\")"=w85) -> ("States Out"=w84:string)  [unwired: 13 in]
          }
          event "Refresh": Value Change {
            # "Refresh graphs with any changes in manipulate data tab\n\nwill also display the data in the 'original cond' graph if no\nnew data has been loaded since starting the program"
            n40 = event-data() -> ("OldVal"=w87:bool)  [unwired: 1 in]
            n41 = local write "Refresh"(w87) -> ()
            n42 = call <vilib>:"Add State(s) to Queue__jki_lib_state_machine.vi"("State(s) in Front (\"\")"="UI: Cursor Set >> Busy\nProcess: Manipulate Data\nUI: Cursor Set >> Idle", "State(s) in (\"\")"=w92) -> ("States Out"=w91:string)  [unwired: 13 in]
          }
          event "Flattened Trans": Cursor Move {
            n43 = event-data() -> ()  [unwired: 1 in, 9 out]
            n44 = property on="Flattened Trans" class="IntGraph (strict)"() -> ("Cursor.Cursor Index"=w98:i32, "Cursor.Cursor Plot"=w97:i32)  [unwired: 2 in, 2 out]
            n45 = property on="Transcond Intensity" class="IntGraph (strict)"("Cursor.Cursor Index"=w98, "Cursor.Cursor Plot"=w97) -> ()  [unwired: 2 in, 2 out]
            n46 = call <vilib>:"Add State(s) to Queue__jki_lib_state_machine.vi"("State(s) in (\"\")"=w93) -> ("States Out"=w94:string)  [unwired: 14 in]
          }
          event "Cond intensity": Cursor Move {
            n47 = event-data() -> ()  [unwired: 1 in, 9 out]
            n48 = property on="Cond intensity" class="IntGraph (strict)"() -> ("Cursor.Cursor Index"=w100:i32, "Cursor.Cursor Plot"=w99:i32)  [unwired: 2 in, 2 out]
            n49 = property on="Transcond Intensity" class="IntGraph (strict)"("Cursor.Cursor Index"=w100, "Cursor.Cursor Plot"=w99) -> ()  [unwired: 2 in, 2 out]
            n50 = call <vilib>:"Add State(s) to Queue__jki_lib_state_machine.vi"("State(s) in (\"\")"=w103) -> ("States Out"=w102:string)  [unwired: 14 in]
          }
          event "Transcond Intensity": Cursor Move {
            # "Change visible tab in line cut tab control when the cursor on the transconductance intensity plot is moved\nmoving the vertical cursor shows the vertical line cut, moving the horizontal cursor shows the horizontal line cut"
            n51 = event-data() -> ("CursIdx"=w109:i32, "PlotIdx"=w110:i32)  [unwired: 1 in, 7 out]
            n52 = Unbundle By Name(w113) -> ("cursor index"=w112:i32, "cursor plot"=w111:i32)
            n53 = Not Equal?(x=w112, y=w109) -> (x != y?=w107:bool)
            n54 = Not Equal?(x=w111, y=w110) -> (x != y?=w106:bool)
            n55 = And(x=w107, y=w106) -> (x .and. y?=w105:bool)
            n56 = disable-structure shown="Disabled" {
              disable-tunnel: w105 -> [w117 _]
              frame Disabled {
                n57 = case shown="True" w117 {
                  tunnel: [T8."vertical line cut" ("Tab Control 2") T8."Horizontal line cut" ("Tab Control 2")] -> w116
                  frame False {
                  }
                  frame True {
                  }
                }
                n58 = local write "Tab Control 2"(w116) -> ()
              }
              frame Enabled {
              }
            }
            n59 = call <vilib>:"Add State(s) to Queue__jki_lib_state_machine.vi"("State(s) in (\"\")"=w115) -> ("States Out"=w114:string)  [unwired: 14 in]
          }
          event "Export igor files": Value Change {
            n60 = event-data() -> ()  [unwired: 1 in, 6 out]
            n61 = call <vilib>:"Add State(s) to Queue__jki_lib_state_machine.vi"("State(s) in (\"\")"=w122, "State(s) at Back (\"\")"="UI: Cursor Set >> Busy\nProcess: Export to igor\nUI: Cursor Set >> Idle" ("State(s) at Back (\"\")")) -> ("States Out"=w121:string)  [unwired: 13 in]
          }
          event Panel Close? {
            # "Discard the event because we'll close the front panel ourselves in Macro: Exit"
            # "Close Panel button (pressed) Event\n(this executes Macro: Exit to terminate the VI)"
            n62 = event-data() -> ()  [unwired: 1 in, 1 out]
            n63 = call <vilib>:"Add State(s) to Queue__jki_lib_state_machine.vi"("State(s) in Front (\"\")"="Macro: Exit", "State(s) in (\"\")"=w130) -> ("States Out"=w129:string)  [unwired: 13 in]
            n64 = event-data("Discard?"=TRUE) -> ()  [unwired: 1 in, 1 out]
          }
        }
      }
      frame "---------- Core ----------" {
        # "Do not put any code in this frame.\n(it is a separator no-op)"
        n65 = call <vilib>:"Add State(s) to Queue__jki_lib_state_machine.vi"("State(s) in (\"\")"=w134) -> ("States Out"=w133:string)  [unwired: 14 in]
      }
      frame Default {
        w144 = 42 items=["No error", "Argument error", "Memory is full", "Out of zone", "End of file", "File already open", "Generic file I/O error", "File not found", "File permission error", "Disk is full", "Duplicate path", "Too many files open", "System feature not enabled", "Resource file not found", "Cannot add resource", "Resource not found", "Image not found", "Image memory error", "Pen does not exist", "Config type invalid", "Config token not found", "Config parse error", "Config memory error", "Bad external code format", "Bad external code offset", "External code not present", "Null window", "Destroy window error", "Null menu", "Print aborted", "Bad print record", "Print driver error", "Windows error during printing", "Memory error during printing", "Print dialog error", "Generic print error", "Invalid device refnum", "Device not found", "Device parameter error", "Device unit error", "Cannot open device", "Device call aborted", "Generic error", "Cancelled by user", "Object ID too low", "Object ID too high", "Object not in heap", "Unknown heap", "Unknown object (invalid DefProc)", "Unknown object (DefProc not in table)", "Message out of range", "Invalid (null) method", "Unknown message", "Manager call not supported", "Bad address", "Network operation in progress", "Network operation timed out", "Connection is busy", "Network attribute not supported", "Network error", "Address in use", "System out of memory", "Connection aborted", "Connection refused", "Not connected", "Already connected", "Connection closed", "Initialization error (interapplication manager)", "Bad occurrence", "Wait on unbound occurrence handler", "Occurrence queue overflow", "Datalog type conflict", "Unused", "Unrecognized type (interapplication manager)", "Memory corrupt", "Failed to make temporary DLL", "Old CIN version", "Drag socket not found", "Failed to load drop-object", "Failed to register OLE object", "Failed to release OLE object", "Format specifier type mismatch", "Unknown format specifier", "Too few format specifiers", "Too many format specifiers", "Scan failed", "Newer CIN version", "Error converting to variant", "Runtime menu error", "Password tampered", "Variant attribute not found", "Incompatible variant data type", "Event data is not available", "Event Store is not present", "Occurrence is not found", "Event Queue is not created", "Event info is not available", "Refnum passed is NULL", "Error retrieving Class GUID", "Error retrieving CoClass GUID", "Error retrieving TypeLib GUID.", "Bad built application magic bytes.", "Specific driver is different from the specific driver associated with the Logical Name.", "There is no session opened to the class driver.", "Max Error", "MAX - Error with config objects", "MAX - Error loading configuration", "MAX - Group not supported"]
        # "Current State"
        # "Do not delete, rename, or modify this frame.\n(this is used to capture unhandled states and typos)"
        # "Handle mistyped state name (developer tool)"
        n66 = Format Into String(format string="Software Exception: Unhandled State \"%s\"." ("message"), error in=w140, w135) -> (resulting string=w143:string, error out=w142:errorcluster)  [unwired: 1 in]
        n67 = call <vilib>:"Error Cluster From Error Code.vi"("show call chain? (False)"=TRUE, "error in (no error)"=w142, "error message (\"\")"=w143, "error code (0)"=w144) -> ("error out"=w141:errorcluster)  [unwired: 5 in]
        n68 = call <vilib>:"Add State(s) to Queue__jki_lib_state_machine.vi"("State(s) in (\"\")"=w139) -> ("States Out"=w138:string)  [unwired: 14 in]
      }
      frame "Initialize Core Data" {
        # "Do not delete, rename, or modify this frame.\n(this is used to determine panel behavior on exit)"
        # "originally closed?"
        # "exe?"
        # "If panel starts closed or is an EXE, then close it when we exit"
        n69 = property class="VI"() -> ("Front Panel.Open"=w153:bool)  [unwired: 2 in, 2 out]
        n70 = property class="App"() -> ("App.Kind"=w152:T9)  [unwired: 2 in, 2 out]
        n71 = control-ref of="Current VI Reference"() -> (w146:refnum<vi>)
        n72 = Not(x=w153) -> (.not. x?=w150:bool)
        n73 = Equal?(x=w152, y=T9."Run Time System" ("Application:Kind")) -> (x = y?=w149:bool)
        n74 = Or(x=w150, y=w149) -> (x .or. y?=w147:bool)
        n75 = Bundle By Name(cluster=w148, "Core.Current VI Reference"=w146, "Core.Close Panel on Exit?"=w147) -> (w155:T14)
        n76 = call <vilib>:"Add State(s) to Queue__jki_lib_state_machine.vi"("State(s) in (\"\")"=w157) -> ("States Out"=w156:string)  [unwired: 14 in]
      }
      frame "Error Handler" {
        # "Unhandled Error -- Display it"
        # "Handle any errors here.\nYou can also output any states to clean-up after errors occur"
        # "Clear error"
        n77 = call <vilib>:"General Error Handler.vi"("error in (no error)"=w159) -> ()  [unwired: 10 in, 5 out]
        n78 = call <vilib>:"Add State(s) to Queue__jki_lib_state_machine.vi"("State(s) in Front (\"\")"="/* Post Error States", "State(s) in (\"\")"=w163) -> ("States Out"=w162:string)  [unwired: 13 in]
      }
      frame "Exit" {
        # "Do not put any code in this frame.\n(No errors that occur here will be handled.)"
        n79 = call <vilib>:"Add State(s) to Queue__jki_lib_state_machine.vi"("State(s) in (\"\")"=w168) -> ("States Out"=w167:string)  [unwired: 14 in]
      }
      frame "---------- Data ----------" {
        # "Do not put any code in this frame.\n(It is a separator no-op. You can make a copy of this frame to create a new Data frame)"
        n80 = call <vilib>:"Add State(s) to Queue__jki_lib_state_machine.vi"("State(s) in (\"\")"=w172) -> ("States Out"=w171:string)  [unwired: 14 in]
      }
      frame "Data: Initialize" {
        w174 = T15 {"ITX File or Folder Path"=path "", "Blob File Path"=path ""}  # Config Cluster
        w178 = refnum<class "Configuration.lvclass"> refnum  # Configuration
        w175 = 0  # resample index
        w176 = 0  # cursor index
        w177 = 0  # cursor plot
        w180 = T4 []  # Modified Transconductance
        w181 = 0  # number of curves
        w182 = cluster{dbl, dbl} {0.0, 0.0}  # B offset and mult
        w183 = cluster{dbl, dbl} {0.0, 0.0}  # Vsg offset and mult
        w184 = dbl[] []  # N1 (B field)
        w185 = T4 []  # Modified Conductance
        w186 = T16 [{"N1"=0.1054, "N2"=0.0, "N3"=7.167371706088133e-06, "N4"=1.53337376832391e-06}, {"N1"=0.2744, "N2"=0.0, "N3"=7.516017465840743e-06, "N4"=1.870780961155766e-06}, {"N1"=0.4429, "N2"=0.0, "N3"=7.164956665698316e-06, "N4"=2.24365763977575e-06}, {"N1"=0.6118, "N2"=0.0, "N3"=7.47503008732585e-06, "N4"=2.509786953376164e-06}, {"N1"=0.78, "N2"=0.0, "N3"=7.582119269367365e-06, "N4"=1.865776048611999e-06}, {"N1"=0.9496, "N2"=0.0, "N3"=7.367991857506643e-06, "N4"=2.698521756661702e-06}, {"N1"=1.1176, "N2"=0.0, "N3"=7.227789507339006e-06, "N4"=2.57461130832219e-06}, {"N1"=1.2843, "N2"=0.0, "N3"=7.066841533109455e-06, "N4"=3.048492296414582e-06}, {"N1"=1.4544, "N2"=0.0, "N3"=6.956050970108828e-06, "N4"=3.922270862071821e-06}, {"N1"=1.6231, "N2"=0.0, "N3"=7.236120895401367e-06, "N4"=3.382292471609201e-06}, {"N1"=1.7923, "N2"=0.0, "N3"=7.409928531135188e-06, "N4"=2.980502224034656e-06}, {"N1"=1.9608, "N2"=0.0, "N3"=7.465240274926555e-06, "N4"=2.567980193012299e-06}, {"N1"=2.1296, "N2"=0.0, "N3"=7.67996705698243e-06, "N4"=2.820594776222847e-06}, {"N1"=2.2974, "N2"=0.0, "N3"=7.462806473700619e-06, "N4"=3.043330294253364e-06}, {"N1"=2.4668, "N2"=0.0, "N3"=7.436808347763807e-06, "N4"=2.755707470732885e-06}, {"N1"=2.6348, "N2"=0.0, "N3"=6.62119487806683e-06, "N4"=3.938204565752024e-06}, {"N1"=2.8044, "N2"=0.0, "N3"=7.474110207381518e-06, "N4"=2.685132266272008e-06}, {"N1"=2.9727, "N2"=0.0, "N3"=7.467721317681889e-06, "N4"=2.490711666292731e-06}, {"N1"=3.1413, "N2"=0.0, "N3"=7.373756967263423e-06, "N4"=3.233877080828954e-06}, {"N1"=3.3108, "N2"=0.0, "N3"=7.665479000670658e-06, "N4"=2.656474229977507e-06}, {"N1"=3.4787, "N2"=0.0, "N3"=7.590986063837561e-06, "N4"=2.372468698283599e-06}, {"N1"=3.6474, "N2"=0.0, "N3"=7.403426727936138e-06, "N4"=2.492719733694041e-06}, {"N1"=3.8169, "N2"=0.0, "N3"=7.673375229594714e-06, "N4"=2.203309425429715e-06}, {"N1"=3.9853, "N2"=0.0, "N3"=7.235339121315365e-06, "N4"=2.455197981754483e-06}, {"N1"=4.1517, "N2"=0.0, "N3"=7.588783683002382e-06, "N4"=2.171945449692774e-06}, {"N1"=4.3221, "N2"=0.0, "N3"=7.448410925151985e-06, "N4"=2.89278994654584e-06}, {"N1"=4.4909, "N2"=0.0, "N3"=7.559811002403063e-06, "N4"=2.32906566750442e-06}, {"N1"=4.6597, "N2"=0.0, "N3"=7.589944875648538e-06, "N4"=2.522315779577562e-06}, {"N1"=4.828, "N2"=0.0, "N3"=7.486560787096485e-06, "N4"=2.673968837700548e-06}, {"N1"=4.9975, "N2"=0.0, "N3"=7.764068992589737e-06, "N4"=2.470810112270278e-06}, {"N1"=5.1656, "N2"=0.0, "N3"=7.515430091426793e-06, "N4"=2.347750168384078e-06}, {"N1"=5.3343, "N2"=0.0, "N3"=7.61778177581086e-06, "N4"=2.441280739349988e-06}, {"N1"=5.5028, "N2"=0.0, "N3"=7.648092365254961e-06, "N4"=2.50884391552613e-06}, {"N1"=5.6718, "N2"=0.0, "N3"=7.607187802074639e-06, "N4"=2.479224506195392e-06}, {"N1"=5.8408, "N2"=0.0, "N3"=7.675790190344634e-06, "N4"=2.243726367409315e-06}, {"N1"=6.0093, "N2"=0.0, "N3"=7.5989905280867e-06, "N4"=2.339493694595715e-06}, {"N1"=6.1776, "N2"=0.0, "N3"=7.946377320613181e-06, "N4"=2.179171604450671e-06}, {"N1"=6.3464, "N2"=0.0, "N3"=7.788145582711778e-06, "N4"=1.980962373666305e-06}, {"N1"=6.5143, "N2"=0.0, "N3"=7.613597487476077e-06, "N4"=2.305590643717492e-06}, {"N1"=6.6841, "N2"=0.0, "N3"=7.704173394418159e-06, "N4"=2.229928539054291e-06}, {"N1"=6.8524, "N2"=0.0, "N3"=7.719187746028896e-06, "N4"=1.959910122360407e-06}, {"N1"=7.0199, "N2"=0.0, "N3"=7.54069778807839e-06, "N4"=2.119395007811887e-06}, {"N1"=7.1892, "N2"=0.0, "N3"=7.780578976603794e-06, "N4"=2.065252716472169e-06}, {"N1"=7.359, "N2"=0.0, "N3"=7.850755995736213e-06, "N4"=2.026777225217505e-06}, {"N1"=7.5271, "N2"=0.0, "N3"=7.948557406193015e-06, "N4"=2.288103766199132e-06}, {"N1"=7.6959, "N2"=0.0, "N3"=7.516853899196371e-06, "N4"=1.934437391177251e-06}, {"N1"=7.8642, "N2"=0.0, "N3"=7.636061465147594e-06, "N4"=2.309715289559359e-06}, {"N1"=8.0328, "N2"=0.0, "N3"=7.633733901431548e-06, "N4"=2.130290776686087e-06}, {"N1"=8.2016, "N2"=0.0, "N3"=7.731748664793311e-06, "N4"=2.089276305545186e-06}, {"N1"=8.3703, "N2"=0.0, "N3"=7.724840467667309e-06, "N4"=2.368731238393298e-06}, {"N1"=8.5396, "N2"=0.0, "N3"=7.765278384713542e-06, "N4"=1.945694195098239e-06}, {"N1"=8.7073, "N2"=0.0, "N3"=7.74873723912328e-06, "N4"=2.207113540673977e-06}, {"N1"=8.8765, "N2"=0.0, "N3"=7.855372955985145e-06, "N4"=1.962585706208197e-06}, {"N1"=9.0455, "N2"=0.0, "N3"=7.843310241373774e-06, "N4"=1.925552700333144e-06}, {"N1"=9.2141, "N2"=0.0, "N3"=7.86110382470724e-06, "N4"=2.081739111499381e-06}, {"N1"=9.3828, "N2"=0.0, "N3"=7.872060865040445e-06, "N4"=2.103890420690471e-06}, {"N1"=9.5511, "N2"=0.0, "N3"=7.577362880483975e-06, "N4"=3.032802004782522e-06}, {"N1"=9.7204, "N2"=0.0, "N3"=7.687842862590589e-06, "N4"=1.874148578396659e-06}, {"N1"=9.8887, "N2"=0.0, "N3"=8.061821348792517e-06, "N4"=1.394385993232741e-06}, {"N1"=10.0569, "N2"=0.0, "N3"=7.583223692545615e-06, "N4"=1.697687019205293e-06}, {"N1"=10.2263, "N2"=0.0, "N3"=7.959425651648591e-06, "N4"=1.719530895423454e-06}, {"N1"=10.3947, "N2"=0.0, "N3"=8.104826950424347e-06, "N4"=2.217009600034041e-06}, {"N1"=10.5631, "N2"=0.0, "N3"=8.092309435913141e-06, "N4"=1.86506523651042e-06}, {"N1"=10.7318, "N2"=0.0, "N3"=7.8911784041579e-06, "N4"=1.760112429967946e-06}, {"N1"=10.9009, "N2"=0.0, "N3"=7.96909852408623e-06, "N4"=1.66698686793123e-06}, {"N1"=11.0691, "N2"=0.0, "N3"=8.065608528600414e-06, "N4"=1.725471834153319e-06}, {"N1"=11.2379, "N2"=0.0, "N3"=8.155864753688254e-06, "N4"=4.665050563001727e-07}, {"N1"=11.407, "N2"=0.0, "N3"=7.80706842968668e-06, "N4"=1.460679749566241e-06}, {"N1"=11.5756, "N2"=0.0, "N3"=8.12897937207956e-06, "N4"=1.587939803265357e-06}, {"N1"=11.741, "N2"=0.0, "N3"=8.27251103469089e-06, "N4"=1.252388215033951e-06}, {"N1"=11.9126, "N2"=0.0, "N3"=7.797849423968604e-06, "N4"=1.267926363181601e-06}, {"N1"=12.0812, "N2"=0.0, "N3"=8.365431522458954e-06, "N4"=2.092208615272172e-09}, {"N1"=12.2499, "N2"=0.0, "N3"=8.039080769849434e-06, "N4"=9.836766439170422e-07}, {"N1"=12.4185, "N2"=0.0, "N3"=7.907582712890951e-06, "N4"=8.989608522161535e-07}, {"N1"=12.5874, "N2"=0.0, "N3"=8.274090537851438e-06, "N4"=9.664113986898211e-07}, {"N1"=12.756, "N2"=0.0, "N3"=7.839858031313029e-06, "N4"=6.065212034273762e-07}, {"N1"=12.9244, "N2"=0.0, "N3"=8.463881119681138e-06, "N4"=-4.136656659107811e-07}, {"N1"=13.0939, "N2"=0.0, "N3"=8.248317658130382e-06, "N4"=3.8802144716701056e-07}, {"N1"=13.2622, "N2"=0.0, "N3"=8.18069446636197e-06, "N4"=4.001100073970894e-07}, {"N1"=13.4308, "N2"=0.0, "N3"=7.946584223789573e-06, "N4"=4.854531765921596e-07}, {"N1"=13.5989, "N2"=0.0, "N3"=8.256171773806876e-06, "N4"=7.718940191013025e-08}, {"N1"=13.7683, "N2"=0.0, "N3"=8.357762676340478e-06, "N4"=-4.766689453610121e-07}, {"N1"=13.9361, "N2"=0.0, "N3"=8.112662582615276e-06, "N4"=4.696250710037667e-08}, {"N1"=14.1046, "N2"=0.0, "N3"=8.277448925942084e-06, "N4"=1.5985023049004504e-07}, {"N1"=14.2741, "N2"=0.0, "N3"=8.336889123617748e-06, "N4"=-2.0452091750021353e-07}, {"N1"=14.4421, "N2"=0.0, "N3"=8.30998027275276e-06, "N4"=4.5720936631723534e-08}, {"N1"=14.6088, "N2"=0.0, "N3"=8.29428838756584e-06, "N4"=-6.505469695250185e-07}, {"N1"=14.7799, "N2"=0.0, "N3"=8.385821104349947e-06, "N4"=-1.3494022655079468e-07}, {"N1"=14.9477, "N2"=0.0, "N3"=8.153057627152194e-06, "N4"=-3.459524396899026e-07}, {"N1"=15.1168, "N2"=0.0, "N3"=8.227366250614983e-06, "N4"=-1.2248894911569274e-07}, {"N1"=15.2855, "N2"=0.0, "N3"=8.445291874318747e-06, "N4"=-3.92114080863001e-07}, {"N1"=15.4543, "N2"=0.0, "N3"=8.32471765192864e-06, "N4"=-5.0620283647846016e-08}, {"N1"=15.6228, "N2"=0.0, "N3"=8.527397645132e-06, "N4"=-8.537202873107685e-07}, {"N1"=15.7909, "N2"=0.0, "N3"=8.397769046079376e-06, "N4"=-8.032897159765025e-07}, {"N1"=15.9596, "N2"=0.0, "N3"=8.548282390442658e-06, "N4"=-7.548173180977796e-07}, {"N1"=16.1276, "N2"=0.0, "N3"=8.419128550887185e-06, "N4"=-7.633414405502411e-07}, {"N1"=16.2972, "N2"=0.0, "N3"=8.415501486100044e-06, "N4"=-1.285585105550623e-06}, {"N1"=16.4645, "N2"=0.0, "N3"=8.600954461689525e-06, "N4"=-1.312315767726753e-06}, {"N1"=16.6337, "N2"=0.0, "N3"=8.593219192247852e-06, "N4"=-9.612729610059892e-07}, {"N1"=16.8019, "N2"=0.0, "N3"=8.389546202306117e-06, "N4"=-9.411302314844897e-07}, {"N1"=16.9709, "N2"=0.0, "N3"=8.71566870861619e-06, "N4"=-1.17801856081449e-06}, {"N1"=17.1383, "N2"=0.0, "N3"=8.425705561859544e-06, "N4"=-1.128343590270702e-06}, {"N1"=17.3074, "N2"=0.0, "N3"=8.712433922967295e-06, "N4"=-1.49946252612336e-06}, {"N1"=17.4742, "N2"=0.0, "N3"=8.790090932572884e-06, "N4"=-1.346827964006174e-06}, {"N1"=17.6436, "N2"=0.0, "N3"=8.704668257768896e-06, "N4"=-1.270644334526553e-06}, {"N1"=17.812, "N2"=0.0, "N3"=8.643630301112523e-06, "N4"=-1.240804614481721e-06}, {"N1"=17.9808, "N2"=0.0, "N3"=8.593810256963035e-06, "N4"=-1.493504631387627e-06}, {"N1"=18.0004, "N2"=0.0, "N3"=8.77741280386506e-06, "N4"=-1.330698644381706e-06}]  # N Array
        w187 = dbl[][] []  # Transcond Intensity
        w188 = dbl[][] []  # Cond Intensity
        w189 = T4 []  # Transconductance
        w190 = T4 []  # Original Conductance
        w191 = T17 {"Current VI Reference"=refnum, "Close Panel on Exit?"=FALSE}  # Core
        # "Initialize the shift-register data, here.\n(data names are defined by what you wire into the bundle function)"
        n81 = call <vilib>:"Add State(s) to Queue__jki_lib_state_machine.vi"("State(s) in (\"\")"=w194) -> ("States Out"=w193:string)  [unwired: 14 in]
        n82 = Bundle("Core"=w191, "Original Conductance"=w190, "Modified Conductance"=w185, "Transconductance"=w189, "Modified Transconductance"=w180, "Cond Intensity"=w188, "Transcond Intensity"=w187, "N Array"=w186, "N1 (B field)"=w184, "Vsg offset and mult"=w183, "B offset and mult"=w182, "number of curves"=w181, "cursor plot"=w177, "cursor index"=w176, "resample index"=w175, "Configuration"=w178, "Config Cluster"=w174, "TDMS Path"="TDMS Path") -> (w179:T14)  [unwired: 1 in]
      }
      frame "Data: Initialize Config File" {
        w198 = T18 6 items=["User Home"=0, "User Desktop"=1, "User Documents"=2, "User Application Data"=3, "User Preferences"=4, "User Temporary"=5, "Public Documents"=6, "Public Application Data"=7, "Public Preferences"=8, "Public Cache"=13, "System Core Libraries"=9, "System Installed Libraries"=10, "Application Files"=11, "Boot Volume Root"=12] ("system directory type")
        # "Do not put any code in this frame.\n(It is a separator no-op. You can make a copy of this frame to create a new Data frame)"
        n83 = Unbundle By Name(w204) -> ("Configuration"=w201:refnum<class "Configuration.lvclass">)
        n84 = call <vilib>:"Get System Directory.vi"("system directory type"=w198) -> ("system directory"=w197:path)  [unwired: 10 in]
        n85 = Build Path(base path=w197, name or relative path="LevyLab\\Process: Transconductance") -> (appended path=w196:path)
        n86 = call-dynamic "Write Path.vi"("error in (no error)"=w200, "Path"=w196, "Configuration in"=w201) -> ("error out"=w199:errorcluster, "Configuration out"=w202:refnum<class "Configuration.lvclass">)  [unwired: 7 in]
        n87 = Bundle By Name(cluster=w204, "Configuration"=w202) -> (w203:T14)
        n88 = call <vilib>:"Add State(s) to Queue__jki_lib_state_machine.vi"("State(s) in (\"\")"=w206) -> ("States Out"=w205:string)  [unwired: 14 in]
      }
      frame "Data: Read Config File" {
        # "Do not put any code in this frame.\n(It is a separator no-op. You can make a copy of this frame to create a new Data frame)"
        n89 = Unbundle By Name(w216) -> ("Config Cluster"=w207:T15, "Configuration"=w218:refnum<class "Configuration.lvclass">)
        n90 = call <userlib>:"Read Configuration.vi"("INI Fomatted Cluster Type"=w207, "error in (no error)"=w214, "Configuration in"=w218) -> ("error out"=w212:errorcluster, "Configuration"=w213:variant, "Configuration out"=w217:refnum<class "Configuration.lvclass">)  [unwired: 6 in]
        n91 = Variant To Data(error in=w212, type=w207, Variant=w213) -> (data=w210:T15, error out=w211:errorcluster)
        n92 = Unbundle By Name(w210) -> ("ITX File or Folder Path"=w209:path, "Blob File Path"=w208:path)
        n93 = Bundle By Name(cluster=w216, "Configuration"=w217) -> (w215:T14)
        n94 = local write "Blob File Path"(w208) -> ()
        n95 = local write "ITX File or Folder Path"(w209) -> ()
        n96 = call <vilib>:"Add State(s) to Queue__jki_lib_state_machine.vi"("State(s) in (\"\")"=w220) -> ("States Out"=w219:string)  [unwired: 14 in]
      }
      frame "Data: Write Config File" {
        # "Do not put any code in this frame.\n(It is a separator no-op. You can make a copy of this frame to create a new Data frame)"
        n97 = local read "Blob File Path"() -> (w222:path)
        n98 = local read "ITX File or Folder Path"() -> (w223:path)
        n99 = Unbundle By Name(w230) -> ("Configuration"=w227:refnum<class "Configuration.lvclass">, "Config Cluster"=w224:T15)
        n100 = Bundle By Name(cluster=w224, "ITX File or Folder Path"=w223, "Blob File Path"=w222) -> (w221:T15)
        n101 = call <userlib>:"Write Configuration.vi"("error in (no error)"=w226, "Variant"=w221, "Configuration in"=w227) -> ("error out"=w225:errorcluster, "Configuration out"=w228:refnum<class "Configuration.lvclass">)  [unwired: 7 in]
        n102 = Bundle By Name(cluster=w230, "Configuration"=w228) -> (w229:T14)
        n103 = call <vilib>:"Add State(s) to Queue__jki_lib_state_machine.vi"("State(s) in (\"\")"=w232) -> ("States Out"=w231:string)  [unwired: 14 in]
      }
      frame "Data: Cleanup" {
        # "Cleanup any data and references, here.\n(this is called automatically, by the Macro: Exit)"
        n104 = Unbundle By Name(w233) -> ("Core.Current VI Reference"=w236:refnum<vi>)
        n105 = Close Reference(reference=w236, error in (no error)=w235) -> (error out=w234:errorcluster)
        n106 = call <vilib>:"Add State(s) to Queue__jki_lib_state_machine.vi"("State(s) in (\"\")"=w238) -> ("States Out"=w237:string)  [unwired: 14 in]
      }
      frame "---------- UI ----------" {
        # "Do not put any code in this frame.\n(It is a separator no-op. You can make a copy of this frame to create a new UI frame)"
        n107 = call <vilib>:"Add State(s) to Queue__jki_lib_state_machine.vi"("State(s) in (\"\")"=w242) -> ("States Out"=w241:string)  [unwired: 14 in]
      }
      frame "UI: Initialize" {
        n108 = local read "Conductance vs Vsg"() -> (w257:cluster{"N1 (B field)":dbl[], dbl[]}[])
        n109 = local read "B Field Array"() -> (w253:dbl[])
        n110 = property on="Transcond Intensity" class="IntGraph (strict)"() -> ("YScale.Ofst&Mult"=w254:T19)  [unwired: 2 in, 2 out]
        n111 = property on="Transcond Intensity" class="IntGraph (strict)"() -> ("XScale.Ofst&Mult"=w255:T19)  [unwired: 2 in, 2 out]
        n112 = local read "horizontal line cut\ncursor index"() -> (w252:i32)
        n113 = control-ref of="Read ITX Data"() -> (w249:refnum<vi>)
        n114 = control-ref of="Resample"() -> (w248:refnum<vi>)
        n115 = control-ref of="Read Blob Data"() -> (w247:refnum<vi>)
        n116 = control-ref of="Refresh"() -> (w246:refnum<vi>)
        n117 = control-ref of="Stop"() -> (w245:refnum<vi>)
        n118 = control-ref of="Clear Graphs & Stop"() -> (w244:refnum<vi>)
        n119 = Build Array(w249, w248, w247, w246, w245, w244) -> (w243:refnum<vi>[])
        n120 = for {
          tunnel: w243 -> [w262] mode=indexing
          n121 = property class="Bool (strict)"(reference=w262, "Value"=FALSE) -> ()  [unwired: 1 in, 2 out]
        }
        n122 = Bundle By Name(cluster=w258, "Original Conductance"=w257, "Vsg offset and mult"=w254, "B offset and mult"=w255, "N1 (B field)"=w253, "resample index"=w252) -> (w256:T14)
        n123 = call <userlib>:"Fit VI window to Content__ogtk.vi"("error in (no error)"=w251) -> ("error out"=w250:errorcluster)  [unwired: 5 in, 1 out]
        n124 = call <vilib>:"Add State(s) to Queue__jki_lib_state_machine.vi"("State(s) in (\"\")"=w260) -> ("States Out"=w259:string)  [unwired: 14 in]
      }
      frame "UI: Cleanup" {
        # "Do not put any code in this frame.\n(It is a separator no-op. You can make a copy of this frame to create a new UI frame)"
        n125 = control-ref of="Read ITX Data"() -> (w269:refnum<vi>)
        n126 = control-ref of="Resample"() -> (w268:refnum<vi>)
        n127 = control-ref of="Read Blob Data"() -> (w267:refnum<vi>)
        n128 = control-ref of="Refresh"() -> (w266:refnum<vi>)
        n129 = control-ref of="Stop"() -> (w265:refnum<vi>)
        n130 = control-ref of="Clear Graphs & Stop"() -> (w264:refnum<vi>)
        n131 = Build Array(w269, w268, w267, w266, w265, w264) -> (w263:refnum<vi>[])
        n132 = for {
          tunnel: w263 -> [w275] mode=indexing
          n133 = property class="Bool (strict)"(reference=w275, "Value"=FALSE) -> ()  [unwired: 1 in, 2 out]
        }
        n134 = call <vilib>:"Add State(s) to Queue__jki_lib_state_machine.vi"("State(s) in (\"\")"=w273) -> ("States Out"=w272:string)  [unwired: 14 in]
      }
      frame "UI: Cursor Set" {
        # "Argument"
        # "Set and Unset Cursor Busy.\n(Usage: \"UI: Cursor Set >> Busy|Idle\")"
        n135 = case shown="\"Busy\"" w276 {
          tunnel: w278 -> [w283 w285]
          tunnel: [w282 w284] -> w277
          frame "Idle", Default {
            n136 = call <vilib>:"Unset Busy.vi"("error in (no error)"=w283) -> ("error out"=w282:errorcluster)  [unwired: 10 in]
          }
          frame "Busy" {
            n137 = call <vilib>:"Set Busy.vi"("error in (no error)"=w285) -> ("error out"=w284:errorcluster)  [unwired: 9 in, 1 out]
          }
        }
        n138 = call <vilib>:"Add State(s) to Queue__jki_lib_state_machine.vi"("State(s) in (\"\")"=w281) -> ("States Out"=w280:string)  [unwired: 14 in]
      }
      frame "UI: Front Panel State" {
        # "Argument"
        # "Set Front Panel Open or Closed\n(Usage: \"UI: Front Panel State >> Open|Close\")"
        n139 = Unbundle By Name(w288) -> ("Core.Current VI Reference"=w287:refnum<vi>)
        n140 = case shown="\"Open\", Default" w286 {
          tunnel: w290 -> [w296 w309]
          tunnel: [w298 w310] -> w289
          tunnel: w287 -> [w297 w307]
          frame "Open", Default {
            n141 = property class="VI"(reference=w297, error in=w296) -> (reference out=w294:refnum<vi>, error out=w295:errorcluster, "Front Panel.Open"=w293:bool)
            n142 = case shown="False" w293 {
              tunnel: [w301 w304] -> w298
              tunnel: w295 -> [w300 w304]
              tunnel: w294 -> [w299 _]
              frame False {
                n143 = invoke class="VI" method="FP.Open"(reference=w299, error in=w300, "Activate"=TRUE, "State"=T10."Standard") -> (error out=w301:errorcluster)  [unwired: 1 in, 4 out]
              }
              frame True {
              }
            }
          }
          frame "Close" {
            n144 = property class="VI"(reference=w307, error in=w309) -> (reference out=w306:refnum<vi>, error out=w308:errorcluster, "Front Panel.Open"=w305:bool)
            n145 = case shown="True" w305 {
              tunnel: [w311 w314] -> w310
              tunnel: w308 -> [w311 w313]
              tunnel: w306 -> [_ w312]
              frame False {
              }
              frame True {
                n146 = invoke class="VI" method="FP.Close"(reference=w312, error in=w313) -> (error out=w314:errorcluster)  [unwired: 1 in, 2 out]
              }
            }
          }
        }
        n147 = call <vilib>:"Add State(s) to Queue__jki_lib_state_machine.vi"("State(s) in (\"\")"=w292) -> ("States Out"=w291:string)  [unwired: 14 in]
      }
      frame "UI: Clear graphs" {
        n148 = invoke on="Conductance vs Vsg" class="XYGraph (strict)" method="Reinit To Default"() -> ()  [unwired: 3 in, 3 out]
        n149 = invoke on="Cond intensity" class="IntGraph (strict)" method="Reinit To Default"() -> ()  [unwired: 3 in, 3 out]
        n150 = invoke on="Conductance" class="XYGraph (strict)" method="Reinit To Default"() -> ()  [unwired: 3 in, 3 out]
        n151 = invoke on="Transconductance" class="XYGraph (strict)" method="Reinit To Default"() -> ()  [unwired: 3 in, 3 out]
        n152 = invoke on="Transcond Intensity" class="IntGraph (strict)" method="Reinit To Default"() -> ()  [unwired: 3 in, 3 out]
        n153 = invoke on="Flattened Trans" class="IntGraph (strict)" method="Reinit To Default"() -> ()  [unwired: 3 in, 3 out]
        n154 = invoke on="modified trans" class="XYGraph (strict)" method="Reinit To Default"() -> ()  [unwired: 3 in, 3 out]
        n155 = invoke on="Vertical Line Cut" class="XYGraph (strict)" method="Reinit To Default"() -> ()  [unwired: 3 in, 3 out]
        n156 = invoke on="Horizontal Line Cut" class="XYGraph (strict)" method="Reinit To Default"() -> ()  [unwired: 3 in, 3 out]
        n157 = call <vilib>:"Add State(s) to Queue__jki_lib_state_machine.vi"("State(s) in (\"\")"=w316) -> ("States Out"=w315:string)  [unwired: 14 in]
      }
      frame "---------- Macro ----------" {
        # "Do not put any code in this frame.\n(It is a separator no-op. You can make a copy of this frame to create a new Macro frame)"
        n158 = call <vilib>:"Add State(s) to Queue__jki_lib_state_machine.vi"("State(s) in (\"\")"=w322) -> ("States Out"=w321:string)  [unwired: 14 in]
      }
      frame "Macro: Initialize" {
        w323 = "Data: Initialize\nInitialize Core Data\nUI: Initialize\nUI: Front Panel State >> Open\nData: Initialize Config File\nData: Read Config File"  # Data: Initialize Initialize Core Data UI: Initialize UI: Front Panel State >> Open Data: Initialize Config File Data: Read Config File
        # "Initialization Macro\n(This is called once, when the VI starts)"
        n159 = call <vilib>:"Add State(s) to Queue__jki_lib_state_machine.vi"("State(s) in Front (\"\")"=w323, "State(s) in (\"\")"=w327) -> ("States Out"=w326:string)  [unwired: 13 in]
      }
      frame "Macro: Exit" {
        # "Exit Macro\n(This is called once, when the VI exits)"
        n160 = Unbundle By Name(w335) -> ("Core.Close Panel on Exit?"=w334:bool)
        n161 = Select(t="UI: Front Panel State >> Close", s=w334, f="") -> (s? t:f=w331:string)
        n162 = call <vilib>:"Add State(s) to Queue__jki_lib_state_machine.vi"("State(s) in Front (\"\")"="Data: Write Config File\nUI: Cleanup", "State(s) in (\"\")"=w331, "State(s) at Back (\"\")"="Data: Cleanup\nExit") -> ("States Out"=w329:string)  [unwired: 12 in]
        n163 = call <vilib>:"Add State(s) to Queue__jki_lib_state_machine.vi"("State(s) in Front (\"\")"=w329, "State(s) in (\"\")"=w338) -> ("States Out"=w337:string)  [unwired: 13 in]
      }
      frame "---------- Process ----------" {
        # "Template Separator\n(You can make a copy of, or modify, this frame)"
        n164 = call <vilib>:"Add State(s) to Queue__jki_lib_state_machine.vi"("State(s) in (\"\")"=w342) -> ("States Out"=w341:string)  [unwired: 14 in]
      }
      frame "Process: Load ITX Data" {
        # "first and last\nB field values"
        # "get B field array"
        # "reverse arrays if field if it is not rising"
        # "calculate B offset and multiplier\nfor intensity plots"
        # "doesn't work if field is swept \nin multiple directions"
        # "Load conductance data"
        # "calculate Vsg offset and multiplier for intensity plots"
        n165 = local read "ITX File or Folder Path"() -> (w358:path)
        n166 = local read "Indices"() -> (w383:T3)
        n167 = call "Calculate conductance ITX.vi"("single ended?"="single ended?", "progress bar?"=TRUE, "length"="File length", "offset"="File offset", "index"=w383, "File or Folder Path"=w358) -> ("N Array"=w360:T16, "Comments"=→"Notes":string, "A vs D"=w345:cluster{dbl[], dbl[]}[])  [unwired: 3 out]
        n168 = for {
          tunnel: w360 -> [w398] mode=indexing
          tunnel: [w397] -> w353 mode=indexing
          tunnel: [w396] -> w355 mode=indexing
          i -> [w396]
          n169 = Unbundle By Name(w398) -> ("N1"=w397:dbl)
        }
        n170 = Index Array(array=w345) -> (element=w375:cluster{dbl[], dbl[]})  [unwired: 1 in]
        n171 = Array Size(array=w345) -> (size(s)=w361:i32)
        n172 = Unbundle(w375) -> (w378:dbl[])  [unwired: 1 out]
        n173 = Array Size(array=w353) -> (size(s)=w373:i32)
        n174 = Array Max & Min(array=w378) -> (min value=w374:dbl)  [unwired: 3 out]
        n175 = Index Array(array=w378, index #1=1 ("index"), index #2=0 ("index")) -> (element #1=w377:dbl, element #2=w376:dbl)
        n176 = call <vilib>:"Linear Fit.vi"("Y"=w353, "X"=w355) -> ("slope"=w354:dbl)  [unwired: 9 in, 4 out]
        n177 = Decrement(x=w373) -> (x-1=w372:i32)
        n178 = Subtract(x=w377, y=w376) -> (x-y=w357:dbl)
        n179 = Less Than 0?(x=w354) -> (x < 0?=w352:bool)
        n180 = case shown="True" w352 {
          tunnel: w345 -> [w391 w395]
          tunnel: w353 -> [w390 w393]
          tunnel: [w391 w394] -> w344
          tunnel: [w390 w392] -> w348
          frame False {
          }
          frame True {
            n181 = Reverse 1D Array(array=w395) -> (reversed array=w394:cluster{dbl[], dbl[]}[])
            n182 = Reverse 1D Array(array=w393) -> (reversed array=w392:dbl[])
          }
        }
        n183 = Bundle(w374, w357) -> (w362:cluster{dbl, dbl})  [unwired: 1 in]
        n184 = case shown="False" "B field in T?" {
          tunnel: w348 -> [w387 w389]
          tunnel: [w386 w389] -> w347
          frame False {
            # "convert to tesla from Oe"
            n185 = Divide(x=w387, y=10000.0) -> (x/y=w386:dbl[])
          }
          frame True {
          }
        }
        n186 = Index Array(array=w347, index #1=0 ("index"), index #2=w372) -> (element #1=w369:dbl, element #2=w370:dbl)
        n187 = Subtract(x=w369, y=w370) -> (x-y=w368:dbl)
        n188 = Absolute Value(x=w368) -> (abs(x)=w367:dbl)
        n189 = Divide(x=w367, y=w361) -> (x/y=w346:dbl)
        n190 = Bundle("N1"=w369, w346) -> (w359:cluster{"N1":dbl, dbl})  [unwired: 1 in]
        n191 = local write "B Field Array"(w347) -> ()
        n192 = local write "Conductance vs Vsg"(w344) -> ()
        n193 = local write "Decimation"(1 ("Decimation")) -> ()
        n194 = Bundle By Name(cluster=w366, "Vsg offset and mult"=w362, "number of curves"=w361, "Original Conductance"=w344, "N Array"=w360, "N1 (B field)"=w347, "B offset and mult"=w359) -> (w382:T14)
        n195 = call <vilib>:"Add State(s) to Queue__jki_lib_state_machine.vi"("State(s) in (\"\")"=w385, "State(s) at Back (\"\")"="Process: Manipulate Data" ("State(s) at Back (\"\")")) -> ("States Out"=w384:string)  [unwired: 13 in]
      }
      frame "Process: Load TDMS Data" {
        # "Do not put any code in this frame.\n(it is a separator no-op)"
        n196 = property on="V1" class="Ring (strict)"() -> ("Strings []"=w425:string[])  [unwired: 2 in, 2 out]
        n197 = Unbundle By Name(w409) -> ("TDMS Path"=w418:path)
        n198 = Index Array(array=w425, index #1="V1", index #2="V2", index #3="CURRENT", index #4="Vsg", index #5="B") -> (element #1=w416:string, element #2=w415:string, element #3=w414:string, element #4=w413:string, element #5=w412:string)
        n199 = TDMS Open(8:w405, 11:w418) -> (0:w420:errorcluster, 3:w419:refnum<k34>)  [unwired: 5 in]
        n200 = TDMS List Contents(4:w420, 7:w419) -> (0:w411:errorcluster, 2:w417:string[], 3:w410:refnum<k34>)  [unwired: 1 in, 1 out]
        n201 = for {
          tunnel: w417 -> [_] mode=indexing
          tunnel: w416 -> [w464]
          tunnel: w415 -> [w452]
          tunnel: w414 -> [w451]
          tunnel: w413 -> [w450]
          tunnel: w412 -> [w449]
          tunnel: w411 -> [w429]
          tunnel: w410 -> [w460]
          tunnel: [w444] -> w400 mode=indexing
          tunnel: [w441] -> w402 mode=indexing
          tunnel: [w439] -> w407
          tunnel: [w438] -> w406
          tunnel: [w432] -> w401
          i -> [w431]
          w453 = dbl[] [] ("array type (2D Dbl)")
          n202 = call "Index to TDMS.Group Name.vi"("error in (no error)"=w429, "Append Index"=w431) -> ("error out"=w428:errorcluster, "group name in (Untitled)"=w430:string)  [unwired: 8 in]
          n203 = TDMS Read(0:w460, 5:w430, 7:w464, 11:w428, 12:w453) -> (4:w459:refnum<k34>, 6:w448:string, 10:w435:dbl[], 15:w458:errorcluster)  [unwired: 3 in, 2 out]
          n204 = TDMS Read(0:w459, 5:w448, 7:w452, 11:w458, 12:w453) -> (4:w463:refnum<k34>, 6:w462:string, 10:w434:dbl[], 15:w461:errorcluster)  [unwired: 3 in, 2 out]
          n205 = TDMS Read(0:w463, 5:w462, 7:w451, 11:w461, 12:w453) -> (4:w457:refnum<k34>, 6:w447:string, 10:w437:dbl[], 15:w454:errorcluster)  [unwired: 3 in, 2 out]
          n206 = TDMS Read(0:w457, 5:w447, 7:w450, 11:w454, 12:w453) -> (4:w456:refnum<k34>, 6:w446:string, 10:w433:dbl[], 15:w455:errorcluster)  [unwired: 3 in, 2 out]
          n207 = Subtract(x=w435, y=w434) -> (x-y=w436:dbl[])
          n208 = Divide(x=w437, y=w436) -> (x/y=w443:dbl[])
          n209 = TDMS Read(0:w456, 5:w446, 7:w449, 11:w455, 12:w453) -> (4:w438:refnum<k34>, 10:w445:dbl[], 15:w439:errorcluster)  [unwired: 3 in, 3 out]
          n210 = Divide(x=w443, y=3.874e-05) -> (x/y=w440:dbl[])
          n211 = Index Array(array=w445) -> (element=w444:dbl)  [unwired: 1 in]
          n212 = call "Array to Offset and Multiplier.vi"("Array"=w433) -> ("Offset and Multiplier"=w432:T19)
          n213 = Bundle("array type (2D Dbl)"=w433, w440) -> (w441:cluster{"array type (2D Dbl)":dbl[], dbl[]})  [unwired: 1 in]
        }
        n214 = call <vilib>:"Add State(s) to Queue__jki_lib_state_machine.vi"("State(s) in (\"\")"=w427) -> ("States Out"=w426:string)  [unwired: 14 in]
        n215 = local write "B Field Array"(w400) -> ()
        n216 = call "Array to Offset and Multiplier.vi"("Array"=w400) -> ("Offset and Multiplier"=w399:T19)
        n217 = local write "Conductance vs Vsg"(w402) -> ()
        n218 = TDMS Close(8:w407, 11:w406) -> (0:w404:errorcluster)  [unwired: 1 out]
        n219 = Bundle By Name(cluster=w409, "Original Conductance"=w402, "N1 (B field)"=w400, "Vsg offset and mult"=w401, "B offset and mult"=w399) -> (w408:T14)
      }
      frame "Process: Load TDMS Wavenames" {
        # "Do not put any code in this frame.\n(it is a separator no-op)"
        n220 = Unbundle By Name(w472) -> ("TDMS Path"=w465:path)
        n221 = control-ref of="V1"() -> (w474:refnum<vi>)
        n222 = control-ref of="V2"() -> (w469:refnum<vi>)
        n223 = control-ref of="CURRENT"() -> (w468:refnum<vi>)
        n224 = control-ref of="Vsg"() -> (w467:refnum<vi>)
        n225 = control-ref of="B"() -> (w466:refnum<vi>)
        n226 = Build Array(w474, w469, w468, w467, w466) -> (w473:refnum<vi>[])
        n227 = call <userlib>:"Read TDMS Wavenames into Ring.vi"("error in (no error)"=w471, "Ring Refs []"=w473, "File or Folder Path"=w465) -> ("error out"=w470:errorcluster)  [unwired: 8 in]
        n228 = call <vilib>:"Add State(s) to Queue__jki_lib_state_machine.vi"("State(s) in (\"\")"=w476) -> ("States Out"=w475:string)  [unwired: 14 in]
      }
      frame "Process: Load TDMS Notes" {
        # "Do not put any code in this frame.\n(it is a separator no-op)"
        n229 = Unbundle By Name(w477) -> ("TDMS Path"=w481:path)
        n230 = call <userlib>:"Read TDMS Comments.vi"("error in (no error)"=w478, "path"=w481) -> ("error out"=w480:errorcluster, "Notes"=w479:string)  [unwired: 7 in, 1 out]
        n231 = local write "Notes"(w479) -> ()
        n232 = call <vilib>:"Add State(s) to Queue__jki_lib_state_machine.vi"("State(s) in (\"\")"=w483) -> ("States Out"=w482:string)  [unwired: 14 in]
      }
      frame "Process: Write BLOB" {
        w489 = "," ("name or relative path")
        w491 = "_" ("name or relative path")
        w524 = T20."replace or create" ("operation (0:open)")
        # "create folder and file name for .blob file\nsave in original location, and in a common folder"
        n233 = Unbundle By Name(w513) -> ("Vsg offset and mult"=w512:cluster{dbl, dbl}, "number of curves"=w511:i32, "Original Conductance"=w510:T4, "Modified Conductance"=w509:T4, "N1 (B field)"=w505:dbl[], "B offset and mult"=w504:cluster{dbl, dbl})
        n234 = local read "Indices"() -> (w497:T3)
        n235 = Unbundle By Name(w497) -> ("CURRENT"=w496:i32, "V1"=w495:i32, "V2"=w494:i32)
        n236 = Number To Decimal String(number=w496) -> (decimal integer string=w490:string)  [unwired: 1 in]
        n237 = Number To Decimal String(number=w495) -> (decimal integer string=w488:string)  [unwired: 1 in]
        n238 = Number To Decimal String(number=w494) -> (decimal integer string=w492:string)  [unwired: 1 in]
        n239 = local read "ITX File or Folder Path"() -> (w536:path)
        n240 = case shown="\"modified cond\"" ".blob file \nconductance" {
          tunnel: w510 -> [w540 _]
          tunnel: w509 -> [_ w542]
          tunnel: [w540 w542] -> w508
          tunnel: ["_original" ("name or relative path") "_modified" ("name or relative path")] -> w501
          frame "original cond", Default {
          }
          frame "modified cond" {
          }
        }
        n241 = local read "single ended?"() -> (w487:bool)
        n242 = Concatenate Strings(w491, w490, w489, w488, "-" ("name or relative path"), w492) -> (w485:string)
        n243 = Concatenate Strings(w491, w490, w489, w488) -> (w486:string)
        n244 = local read "Notes"() -> (w503:string)
        n245 = Select(t=w485, s=w487, f=w486) -> (s? t:f=w484:string)
        n246 = Strip Path(path=w536) -> (stripped path=w532:path, name=w499:string)
        n247 = Strip Path(path=w532) -> (name=w533:string)  [unwired: 1 out]
        n248 = Build Path(base path=w532, name or relative path="processed") -> (appended path=w528:path)
        n249 = Concatenate Strings(w533, "_" ("name or relative path"), w499, w501, "blob note", w484, ".blob" ("string")) -> (w535:string)
        n250 = Bundle(cluster=T11 {"Vsg offset and mult"={0.0, 0.0}, "number of curves"=0, "A vs D"=[], "N1 (B field)"=[], "B offset and mult"={"N1"=0.0, 0.0}, "Comments"="IGOR\nX// Date: 2/12/2019 8:21 AM\nX// sweep B=18T to 0T 0.03 T/min\nX// T=26mK\nX// sweep Vsg: -20mV to 40mV, 25uV step\nX// Vbg=-8.7V\nX// lockin settings:\nX// time constant =100ms\nX// order=2\nX// \nX// sampling\nX// Fs=1664\nX// #s=128\nX// \nX// helix\nX// \nX// lockin:\nX// 0: n.c,\nX// 1: 7, current, 50uV AC 405uV DC, 13 Hz\nX// 2: 3, voltage V+\nX// 3: 1, current, drain\nX// 4: 28, voltage V-\nX// 5: 26, voltage V-\nX// 6: n.c,\nX// 7: 5, side gate \nX// \nX// \nX// KH gain 100x\nX// shunt resistor: 50k\nX// `INDEX`<WavesIndex_In_2>\n\nX//   <Side_Gate>1</Side_Gate>\n\nX//   <Current>6</Current>\n\nX//   <Voltage_1>12</Voltage_1>\n\nX//   <Voltage_2>8</Voltage_2>\n\nX//   <B_Field>3</B_Field>\n\nX//   <Voltage>true</Voltage>\n\nX// </WavesIndex_In_2>`INDEX`\n\n\n\n\n\n\n\n\n\n\n\n\n\n\n\n\n\n\n\n\n\n\n\n\n\n\n\n\n\n\n\n\n\n\n\n\n\n\n\n\n\n\n\n\n\n\n\n\n\n\n\n\n\n\n\n\n\n\n\n\n\n\n\n\n\n\nX \nX Display/R 'time.SA03018E.20190209.000260'\nX AppendToGraph 'Vsg.SA03018E.20190209.000260'\nX AppendToGraph 'T.SA03018E.20190209.000260'\nX AppendToGraph 'B.SA03018E.20190209.000260'\nX AppendToGraph 'X0.SA03018E.20190209.000260'\nX AppendToGraph 'Y0.SA03018E.20190209.000260'\nX AppendToGraph 'X1.SA03018E.20190209.000260'\nX AppendToGraph 'Y1.SA03018E.20190209.000260'\nX AppendToGraph 'X2.SA03018E.20190209.000260'\nX AppendToGraph 'Y2.SA03018E.20190209.000260'\nX AppendToGraph 'X3.SA03018E.20190209.000260'\nX AppendToGraph 'Y3.SA03018E.20190209.000260'\nX AppendToGraph 'X4.SA03018E.20190209.000260'\nX AppendToGraph 'Y4.SA03018E.20190209.000260'\nX AppendToGraph 'X5.SA03018E.20190209.000260'\nX AppendToGraph 'Y5.SA03018E.20190209.000260'\nX AppendToGraph 'X6.SA03018E.20190209.000260'\nX AppendToGraph 'Y6.SA03018E.20190209.000260'\nX AppendToGraph 'X7.SA03018E.20190209.000260'\nX AppendToGraph 'Y7.SA03018E.20190209.000260'\nX AppendToGraph 'B_rate.SA03018E.20190209.000260'\nX AppendToGraph 'R4t(e2/h).SA03018E.20190209.000260'\nX AppendToGraph 'axis1.SA03018E.20190209.000260'\nX AppendToGraph 'axis2.SA03018E.20190209.000260'\nX AppendToGraph 'Mean0.SA03018E.20190209.000260'\nX AppendToGraph 'Mean1.SA03018E.20190209.000260'\nX AppendToGraph 'Mean2.SA03018E.20190209.000260'\nX AppendToGraph 'Mean3.SA03018E.20190209.000260'\nX AppendToGraph 'Mean4.SA03018E.20190209.000260'\nX AppendToGraph 'Mean5.SA03018E.20190209.000260'\nX AppendToGraph 'Mean6.SA03018E.20190209.000260'\nX AppendToGraph 'Mean7.SA03018E.20190209.000260'\nX Label bottom \"x label\"\nX Label left \"y label\"\nX ModifyGraph rgb('time.SA03018E.20190209.000260')=(65280,0,0)\nX ModifyGraph rgb('Vsg.SA03018E.20190209.000260')=(65280,10752,0)\nX ModifyGraph rgb('T.SA03018E.20190209.000260')=(65280,21504,0)\nX ModifyGraph rgb('B.SA03018E.20190209.000260')=(65280,33792,0)\nX ModifyGraph rgb('X0.SA03018E.20190209.000260')=(65280,44544,0)\nX ModifyGraph rgb('Y0.SA03018E.20190209.000260')=(65280,55296,0)\nX ModifyGraph rgb('X1.SA03018E.20190209.000260')=(65024,65280,0)\nX ModifyGraph rgb('Y1.SA03018E.20190209.000260')=(54272,65280,0)\nX ModifyGraph rgb('X2.SA03018E.20190209.000260')=(41984,65280,0)\nX ModifyGraph rgb('Y2.SA03018E.20190209.000260')=(31232,65280,0)\nX ModifyGraph rgb('X3.SA03018E.20190209.000260')=(20480,65280,0)\nX ModifyGraph rgb('Y3.SA03018E.20190209.000260')=(9728,65280,0)\nX ModifyGraph rgb('X4.SA03018E.20190209.000260')=(0,65280,1024)\nX ModifyGraph rgb('Y4.SA03018E.20190209.000260')=(0,65280,11776)\nX ModifyGraph rgb('X5.SA03018E.20190209.000260')=(0,65280,24064)\nX ModifyGraph rgb('Y5.SA03018E.20190209.000260')=(0,65280,34816)\nX ModifyGraph rgb('X6.SA03018E.20190209.000260')=(0,65280,45568)\nX ModifyGraph rgb('Y6.SA03018E.20190209.000260')=(0,65280,56320)\nX ModifyGraph rgb('X7.SA03018E.20190209.000260')=(0,64000,65280)\nX ModifyGraph rgb('Y7.SA03018E.20190209.000260')=(0,51712,65280)\nX ModifyGraph rgb('B_rate.SA03018E.20190209.000260')=(0,40960,65280)\nX ModifyGraph rgb('R4t(e2/h).SA03018E.20190209.000260')=(0,30208,65280)\nX ModifyGraph rgb('axis1.SA03018E.20190209.000260')=(0,19456,65280)\nX ModifyGraph rgb('axis2.SA03018E.20190209.000260')=(0,8704,65280)\nX ModifyGraph rgb('Mean0.SA03018E.20190209.000260')=(2048,0,65280)\nX ModifyGraph rgb('Mean1.SA03018E.20190209.000260')=(14336,0,65280)\nX ModifyGraph rgb('Mean2.SA03018E.20190209.000260')=(25088,0,65280)\nX ModifyGraph rgb('Mean3.SA03018E.20190209.000260')=(35840,0,65280)\nX ModifyGraph rgb('Mean4.SA03018E.20190209.000260')=(46592,0,65280)\nX ModifyGraph rgb('Mean5.SA03018E.20190209.000260')=(57344,0,65280)\nX ModifyGraph rgb('Mean6.SA03018E.20190209.000260')=(65280,0,61440)\nX ModifyGraph rgb('Mean7.SA03018E.20190209.000260')=(65280,0,50688)\nX Legend/C/N=text0/J \"\\\\s('time.SA03018E.20190209.000260') time\\r\\\\s('Vsg.SA03018E.20190209.000260') Vsg\\r\\\\s('T.SA03018E.20190209.000260') T\\r\\\\s('B.SA03018E.20190209.000260') B\\r\\\\s('X0.SA03018E.20190209.000260') X0\\r\\\\s('Y0.SA03018E.20190209.000260') Y0\\r\\\\s('X1.SA03018E.20190209.000260') X1\\r\\\\s('Y1.SA03018E.20190209.000260') Y1\\r\\\\s('X2.SA03018E.20190209.000260') X2\\r\\\\s('Y2.SA03018E.20190209.000260') Y2\\r\\\\s('X3.SA03018E.20190209.000260') X3\\r\\\\s('Y3.SA03018E.20190209.000260') Y3\\r\\\\s('X4.SA03018E.20190209.000260') X4\\r\\\\s('Y4.SA03018E.20190209.000260') Y4\\r\\\\s('X5.SA03018E.20190209.000260') X5\\r\\\\s('Y5.SA03018E.20190209.000260') Y5\\r\\\\s('X6.SA03018E.20190209.000260') X6\\r\\\\s('Y6.SA03018E.20190209.000260') Y6\\r\\\\s('X7.SA03018E.20190209.000260') X7\\r\\\\s('Y7.SA03018E.20190209.000260') Y7\\r\\\\s('B_rate.SA03018E.20190209.000260') B_rate\\r\\\\s('R4t(e2/h).SA03018E.20190209.000260') R4t (e2/h)\\r\\\\s('axis1.SA03018E.20190209.000260') axis 1\\r\\\\s('axis2.SA03018E.20190209.000260') axis 2\\r\\\\s('Mean0.SA03018E.20190209.000260') Mean0\\r\\\\s('Mean1.SA03018E.20190209.000260') Mean1\\r\\\\s('Mean2.SA03018E.20190209.000260') Mean2\\r\\\\s('Mean3.SA03018E.20190209.000260') Mean3\\r\\\\s('Mean4.SA03018E.20190209.000260') Mean4\\r\\\\s('Mean5.SA03018E.20190209.000260') Mean5\\r\\\\s('Mean6.SA03018E.20190209.000260') Mean6\\r\\\\s('Mean7.SA03018E.20190209.000260') Mean7\"\nX ModifyGraph mirror(bottom)=1\nX ModifyGraph width=216\nX ModifyGraph height={Aspect,0.6}\nX ModifyGraph Log(bottom)=0\nX ModifyGraph Log(left)=0\nX \n"}, "Vsg offset and mult"=w512, "number of curves"=w511, "A vs D"=w508, "N1 (B field)"=w505, "B offset and mult"=w504, "Comments"=w503) -> (w516:T11)
        n251 = call <userlib>:"Create Dir if Non-Existant__ogtk.vi"("Directory Path"=w528) -> ("dup Directory Path"=w529:path)  [unwired: 8 in, 2 out]
        n252 = call <vilib>:"Add State(s) to Queue__jki_lib_state_machine.vi"("State(s) in (\"\")"=w538) -> ("States Out"=w537:string)  [unwired: 14 in]
        n253 = Build Path(base path=w529, name or relative path=w535) -> (appended path=w525:path)
        n254 = Open/Create/Replace File(file path (use dialog)=w525, error in=w527, operation (0:open)=w524) -> (refnum out=w523:refnum<file>, error out=w521:errorcluster)  [unwired: 3 in, 1 out]
        n255 = Write to Binary File(file (use dialog)=w523, data=w516, error in=w521) -> (refnum out=w522:refnum<file>, error out=w520:errorcluster)  [unwired: 3 in, 1 out]
        n256 = Build Path(base path=path "P:/users1/kirkendall/data/superlattice blob files" ("File or Folder Path"), name or relative path=w535) -> (appended path=w500:path)
        n257 = Close File(refnum=w522, error in=w520) -> (error out=w519:errorcluster)  [unwired: 1 out]
        n258 = Open/Create/Replace File(file path (use dialog)=w500, error in=w519, operation (0:open)=w524) -> (refnum out=w518:refnum<file>, error out=w515:errorcluster)  [unwired: 3 in, 1 out]
        n259 = Write to Binary File(file (use dialog)=w518, data=w516, error in=w515) -> (refnum out=w517:refnum<file>, error out=w514:errorcluster)  [unwired: 3 in, 1 out]
        n260 = Close File(refnum=w517, error in=w514) -> (error out=w526:errorcluster)  [unwired: 1 out]
      }
      frame "Process: Read BLOB" {
        n261 = Read from Binary File(5:T11 {"Vsg offset and mult"={0.0, 0.0}, "number of curves"=0, "A vs D"=[], "N1 (B field)"=[], "B offset and mult"={"N1"=0.0, 0.0}, "Comments"=""} ("cluster"), 8:w546, 11:"Blob File Path") -> (0:w545:errorcluster, 2:w556:T11)  [unwired: 3 in, 2 out]
        n262 = Unbundle By Name(w556) -> ("Vsg offset and mult"=w550:cluster{dbl, dbl}, "number of curves"=w549:i32, "A vs D"=w547:cluster{dbl[], dbl[]}[], "N1 (B field)"=w544:dbl[], "B offset and mult"=w548:cluster{"N1":dbl, dbl}, "Comments"=w551:string)  [unwired: 1 out]
        n263 = local write "Conductance vs Vsg"(w547) -> ()
        n264 = local write "Decimation"(1 ("Decimation")) -> ()
        n265 = local write "Notes"(w551) -> ()
        n266 = local write "B Field Array"(w544) -> ()
        n267 = Bundle By Name(cluster=w553, "Vsg offset and mult"=w550, "number of curves"=w549, "Original Conductance"=w547, "N1 (B field)"=w544, "B offset and mult"=w548) -> (w552:T14)
        n268 = call <vilib>:"Add State(s) to Queue__jki_lib_state_machine.vi"("State(s) in (\"\")"=w559, "State(s) at Back (\"\")"="Process: Manipulate Data" ("State(s) at Back (\"\")")) -> ("States Out"=w558:string)  [unwired: 13 in]
      }
      frame "Process: Manipulate Data" {
        n269 = Unbundle By Name(w569) -> ("Original Conductance"=w575:T4)
        n270 = case shown="True" "restrict range?" {
          tunnel: w575 -> [w597 w603]
          tunnel: [w597 w602] -> w571
          tunnel: w564 -> [w596 w599]
          tunnel: [w596 w598] -> w562
          frame False {
          }
          frame True {
            # "restrict data range"
            n271 = call-poly <userlib>:"Remove Outliers.vi"("error in (no error)"=w599, "Y Lower"="Lower", "Y Upper"="Upper", "XY-data"=w603) -> ("error out"=w598:errorcluster, "XY-data out"=w602:cluster{"X-array":dbl[], "Y-array":dbl[]}[])  [unwired: 6 in]
          }
        }
        n272 = case shown="True" "Filter?" {
          tunnel: w571 -> [w590 w595]
          tunnel: [w590 w594] -> w572
          tunnel: [w589 w592] -> w563
          tunnel: w562 -> [w589 w591]
          frame False {
          }
          frame True {
            # "filter  data"
            n273 = call-poly <userlib>:"Zero Phase Lowpass Filter.vi"("error in (no error)"=w591, "cutoff period"="cutoff period", "XY-data"=w595) -> ("error out"=w592:errorcluster, "XY-data out"=w594:cluster{"X-array":dbl[], "Y-array":dbl[]}[])  [unwired: 7 in]
          }
        }
        n274 = case shown="True" "Multiply" {
          tunnel: w572 -> [w580 w588]
          tunnel: [w580 w583] -> w568
          tunnel: [w579 w582] -> w570
          tunnel: w563 -> [w579 w587]
          frame False {
          }
          frame True {
            n275 = call-poly <userlib>:"Multiply.vi"("error in (no error)"=w587, "x (1)"="alpha", "XY-data"=w588) -> ("error out"=w585:errorcluster, "XY-data out"=w584:cluster{"X-array":dbl[], "Y-array":dbl[]}[])  [unwired: 7 in]
            n276 = call-poly <userlib>:"Subtract.vi"("error in (no error)"=w585, "x (0)"="mu offset", "XY-data"=w584) -> ("error out"=w582:errorcluster, "XY-data out"=w583:cluster{"X-array":dbl[], "Y-array":dbl[]}[])  [unwired: 7 in]
          }
        }
        n277 = Index Array(array=w568) -> (element=w567:cluster{"X-array":dbl[], "Y-array":dbl[]})  [unwired: 1 in]
        n278 = Unbundle(w567) -> ("X-array"=w566:dbl[])  [unwired: 1 out]
        n279 = call "Array to Offset and Multiplier.vi"("Array"=w566) -> ("Offset and Multiplier"=w565:T19)
        n280 = Bundle By Name(cluster=w569, "Modified Conductance"=w568, "Vsg offset and mult"=w565) -> (w574:T14)
        n281 = call <vilib>:"Add State(s) to Queue__jki_lib_state_machine.vi"("State(s) in (\"\")"=w578, "State(s) at Back (\"\")"="Process: Transconductance" ("State(s) at Back (\"\")")) -> ("States Out"=w577:string)  [unwired: 13 in]
      }
      frame "Process: Resample Data" {
        # "or:\n?"
        # "#todo\nreplace with:"
        n282 = Unbundle By Name(w612) -> ("Modified Conductance"=w610:T4, "N1 (B field)"=w607:dbl[], "resample index"=w609:i32)
        n283 = disable-structure shown="Disabled" {
          frame Disabled {
            # "+"
            n284 = call-poly <userlib>:"Resample.vi"() -> ()  [unwired: 10 in, 2 out]
            n285 = call-poly <userlib>:"Shift Zero.vi"() -> ()  [unwired: 10 in, 2 out]
          }
          frame Enabled {
          }
        }
        n286 = call "split and resample.vi"("real zero index"=w609, "B field array"=w607, "cond"=w610) -> ("resampled number of curves"=w606:i32, "new B field\noffset and multiplier"=w605:cluster{"N1":dbl, dbl}, "resampled B"=w604:dbl[], "resampled cond"=w608:T4)  [unwired: 5 in]
        n287 = disable-structure shown="Disabled" {
          frame Disabled {
            n288 = call-poly <userlib>:"Shift Zero.vi"() -> ()  [unwired: 10 in, 2 out]
          }
          frame Enabled {
          }
        }
        n289 = Bundle By Name(cluster=w612, "Modified Conductance"=w608, "N1 (B field)"=w604, "B offset and mult"=w605, "number of curves"=w606) -> (w611:T14)
        n290 = call <vilib>:"Add State(s) to Queue__jki_lib_state_machine.vi"("State(s) in (\"\")"=w616, "State(s) at Back (\"\")"="Process: Transconductance" ("State(s) at Back (\"\")")) -> ("States Out"=w615:string)  [unwired: 13 in]
      }
      frame "Process: Transconductance" {
        n291 = Unbundle By Name(w617) -> ("Modified Conductance"=w624:T4)
        n292 = call-poly <userlib>:"Derivative.vi"("Interval Units"="Interval Units", "error in (no error)"=w622, "Type"="Derivative Type", "Interval"="Interval", "XY-data"=w624) -> ("error out"=w621:errorcluster, "Differential out"=w623:cluster{"X-array":dbl[], "Y-array":dbl[]}[])  [unwired: 4 in, 1 out]
        n293 = Bundle By Name(cluster=w617, "Transconductance"=w623, "Modified Transconductance"=w623) -> (w626:T14)
        n294 = call <vilib>:"Add State(s) to Queue__jki_lib_state_machine.vi"("State(s) in (\"\")"=w628, "State(s) at Back (\"\")"="Flatten Process: Transconductance" ("State(s) at Back (\"\")")) -> ("States Out"=w627:string)  [unwired: 13 in]
      }
      frame "Process: Flatten Transconductance" {
        n295 = Unbundle By Name(w636) -> ("Transconductance"=w633:T4, "Vsg offset and mult"=w634:cluster{dbl, dbl}, "number of curves"=w632:i32)
        n296 = case shown="True" "flatten trans?" {
          tunnel: w634 -> [_ w648]
          tunnel: [w640 w647] -> w630
          tunnel: w633 -> [w640 w646]
          tunnel: w632 -> [_ w645]
          frame False {
          }
          frame True {
            n297 = Initialize Array(0.0 ("element"), w645) -> (w643:dbl[])
            n298 = Add(x=w643, y="manual offset array") -> (x+y=w641:dbl[])
            n299 = for {
              tunnel: w646 -> [w669] mode=indexing
              tunnel: w648 -> [w664]
              tunnel: [w654] -> w647 mode=indexing
              tunnel: w641 -> [w662] mode=indexing
              n300 = Unbundle(w664) -> (w650:dbl)  [unwired: 1 out]
              n301 = Unbundle(w669) -> ("Vfast"=w656:dbl[], "Decimated Array"=w665:dbl[])
              n302 = call <vilib>:"Peak Detector.vi"("peaks/valleys"=enum32{"Peaks", "Valleys"}."Peaks", "width"="width", "threshold"="threshold", "X"=w665) -> ("Locations"=w657:dbl[])  [unwired: 3 in, 4 out]
              n303 = Index Array(array=w657) -> (element=w666:dbl)  [unwired: 1 in]
              n304 = Index Array(array=w656, index=w666) -> (element=w660:dbl)
              n305 = Subtract(x=w656, y=w660) -> (x-y=w663:dbl[])
              n306 = case shown="\"Add manual offset\"" "add manual offset?" {
                tunnel: w663 -> [_ w673 w674]
                tunnel: w662 -> [w671 _ w675]
                tunnel: [w670 w673 w676] -> w661
                tunnel: w656 -> [w672 _ _]
                frame "Only manual offset", Default {
                  n307 = Add(x=w672, y=w671) -> (x+y=w670:dbl[])
                }
                frame "No manual offset" {
                }
                frame "Add manual offset" {
                  n308 = Add(x=w674, y=w675) -> (x+y=w676:dbl[])
                }
              }
              n309 = Bundle By Name(cluster=T12 {"X Low"=0.05, "X High"=0.5, "X Step"=0.01, "Fake Point"=0.05} ("Configure"), "X Low"="X Low", "X High"="X High", "X Step"=w650) -> (w649:T12)
              n310 = Bundle(w661, "Decimated Array"=w665) -> (w655:cluster{dbl[], "Decimated Array":dbl[]})  [unwired: 1 in]
              n311 = call-poly <userlib>:"Interpolate.vi"("Configure"=w649, "XY-data"=w655) -> ("Interpolated XY-data out"=w654:cluster{"X-array":dbl[], "Y-array":dbl[]})  [unwired: 8 in, 1 out]
            }
            "number of curves" <- w645
          }
        }
        n312 = Bundle By Name(cluster=w636, "Modified Transconductance"=w630) -> (w635:T14)
        n313 = call <vilib>:"Add State(s) to Queue__jki_lib_state_machine.vi"("State(s) in (\"\")"=w639, "State(s) at Back (\"\")"="Process: Display data" ("State(s) at Back (\"\")")) -> ("States Out"=w638:string)  [unwired: 13 in]
      }
      frame "Process: Display data" {
        # "horizontal"
        # "vertical"
        # "decimate number of cond curves"
        # "choose B field values to display for cond plot"
        n314 = Unbundle By Name(w682) -> ("Modified Conductance"=w701:T4, "Transconductance"=w679:T4, "Modified Transconductance"=w718:T4, "Vsg offset and mult"=w683:cluster{dbl, dbl}, "B offset and mult"=w677:cluster{dbl, dbl}, "N1 (B field)"=w693:dbl[])
        "modified trans" <- w718
        n315 = property on="Cond intensity" class="IntGraph (strict)"("XScale.Ofst&Mult"=w677) -> ()  [unwired: 2 in, 2 out]
        n316 = property on="Transcond Intensity" class="IntGraph (strict)"("XScale.Ofst&Mult"=w677) -> ()  [unwired: 2 in, 2 out]
        n317 = property on="Cond intensity" class="IntGraph (strict)"("YScale.Ofst&Mult"=w683) -> ()  [unwired: 2 in, 2 out]
        n318 = property on="Transcond Intensity" class="IntGraph (strict)"("YScale.Ofst&Mult"=w683) -> ()  [unwired: 2 in, 2 out]
        n319 = property on="Flattened Trans" class="IntGraph (strict)"("YScale.Ofst&Mult"=w683) -> ()  [unwired: 2 in, 2 out]
        n320 = property on="Transcond Intensity" class="IntGraph (strict)"() -> ("Cursor.Cursor X"=→"B field (T)":dbl)  [unwired: 2 in, 2 out]
        n321 = property on="Transcond Intensity" class="IntGraph (strict)"() -> ("Cursor.Cursor Y"=→"Vsg (V)":dbl)  [unwired: 2 in, 2 out]
        n322 = call "decimate cond.vi"("Offset"="Offset", "B field array"=w693, "Conductance"=w701, "Decimation"="Decimation") -> ("error out"=w684:errorcluster, "decimated B field array"=w692:dbl[], "Decimated conductance"=w691:T4)  [unwired: 5 in]
        n323 = call <vilib>:"Clear Errors.vi"("error in (no error)"=w684) -> ()  [unwired: 5 in, 2 out]
        n324 = for {
          tunnel: w691 -> [w743] mode=indexing
          tunnel: [w741] -> w690 mode=indexing
          i -> [w742]
          # "this part is\napplying offset"
          n325 = Unbundle(w743) -> ("Vfast"=w747:dbl[], "Decimated Array"=w744:dbl[])
          n326 = Multiply(x="offset cond (horizontal)", y=w742) -> (x*y=w746:dbl)
          n327 = Add(x=w747, y=w746) -> (x+y=w745:dbl[])
          n328 = Bundle(w745, "Decimated Array"=w744) -> (w741:cluster{dbl[], "Decimated Array":dbl[]})  [unwired: 1 in]
        }
        n329 = for {
          tunnel: w679 -> [w769] mode=indexing
          tunnel: [w763] -> w709 mode=indexing
          tunnel: [w766] -> w719 mode=indexing
          tunnel: w718 -> [w765] mode=indexing
          tunnel: [w764] -> w688 mode=indexing
          tunnel: w701 -> [w759] mode=indexing
          tunnel: [w758] -> w700 mode=indexing
          i -> [w760]
          # "this part is doing\nXY to 2D array"
          # "this part is\napplying offset"
          n330 = Unbundle(w759) -> ("Decimated Array"=w758:dbl[])  [unwired: 1 out]
          n331 = Unbundle(w765) -> ("Decimated Array"=w764:dbl[])  [unwired: 1 out]
          n332 = Unbundle(w769) -> ("Vfast"=w762:dbl[], "Decimated Array"=w763:dbl[])
          n333 = Multiply(x="offset trans (vertical)", y=w760) -> (x*y=w767:dbl)
          n334 = Add(x=w763, y=w767) -> (x+y=w761:dbl[])
          n335 = Bundle("Vfast"=w762, w761) -> (w766:cluster{"Vfast":dbl[], dbl[]})  [unwired: 1 in]
        }
        "Cond intensity" <- w700
        "Transcond Intensity" <- w709
        n336 = case shown="\"Transconductance\"" "line cut" {
          tunnel: w709 -> [_ w754]
          tunnel: [w751 w754] -> w708
          tunnel: w700 -> [w751 _]
          tunnel: w701 -> [w749 _]
          tunnel: w679 -> [_ w753]
          tunnel: [w749 w753] -> w707
          tunnel: [" G (e^2/h)" "dG/dVsg (arb.)"] -> w680
          frame "Conductance", Default {
          }
          frame "Transconductance" {
          }
        }
        n337 = disable-structure shown="Disabled" {
          frame Disabled {
            n338 = call-poly <userlib>:"Subset.vi"() -> ()  [unwired: 10 in, 2 out]
          }
          frame Enabled {
          }
        }
        n339 = property on="Horizontal Line Cut" class="XYGraph (strict)"("YScale.NameLbl.Text"=w680) -> ()  [unwired: 2 in, 2 out]
        n340 = property on="Vertical Line Cut" class="XYGraph (strict)"("YScale.NameLbl.Text"=w680) -> ()  [unwired: 2 in, 2 out]
        n341 = local write "Transconductance"(w719) -> ()
        n342 = Threshold 1D Array(2:"start B", 3:w692) -> (0:w695:dbl)  [unwired: 1 in]
        n343 = Transpose 2D Array(2D array=w708) -> (transposed array=w716:dbl[][])
        n344 = property on="Transcond Intensity" class="IntGraph (strict)"() -> ("Cursor.Cursor Index"=w681:i32)  [unwired: 2 in, 2 out]
        n345 = Threshold 1D Array(2:"end B", 3:w692) -> (0:w696:dbl)  [unwired: 1 in]
        n346 = Index Array(array=w707, index=w681) -> (element=w717:cluster{"Vfast":dbl[], "Decimated Array":dbl[]})
        n347 = Subtract(x=w696, y=w695) -> (x-y=w694:dbl)
        n348 = case shown="True" "mirror?" {
          tunnel: w688 -> [w722 w730]
          tunnel: [w722 w732] -> w687
          tunnel: w677 -> [_ w725]
          frame False {
          }
          frame True {
            n349 = Unbundle(w725) -> (w726:dbl)  [unwired: 1 out]
            n350 = Transpose 2D Array(2D array=w730) -> (transposed array=w734:dbl[][])
            n351 = for {
              tunnel: w734 -> [w740] mode=indexing
              tunnel: [w739] -> w733 mode=indexing
              n352 = Reverse 1D Array(array=w740) -> (reversed array=w739:dbl[])
            }
            n353 = Bundle("offset"="offset", w726) -> (w723:cluster{"offset":dbl, dbl})  [unwired: 1 in]
            n354 = Transpose 2D Array(2D array=w733) -> (transposed array=w731:dbl[][])
            n355 = property on="Flattened Trans" class="IntGraph (strict)"("XScale.Ofst&Mult"=w723) -> ()  [unwired: 2 in, 2 out]
            n356 = case shown="True" "flip mirror" {
              tunnel: w731 -> [w735 w737]
              tunnel: w730 -> [w736 w738]
              tunnel: [w735 w738] -> w729
              tunnel: [w736 w737] -> w728
              frame False {
              }
              frame True {
              }
            }
            n357 = Build Array (concatenate)(w729, w728) -> (w732:dbl[][])
          }
        }
        "Flattened Trans" <- w687
        n358 = Build Array(w717) -> (→"Vertical Line Cut":T4)
        n359 = Array Subset(array=w690, index=w695, length=w694) -> (w699:cluster{dbl[], "Decimated Array":dbl[]}[])
        n360 = for {
          tunnel: w716 -> [w756] mode=indexing
          tunnel: w693 -> [w757]
          tunnel: [w755] -> w715 mode=indexing
          n361 = Bundle("N1 (B field)"=w757, w756) -> (w755:cluster{"N1 (B field)":dbl[], dbl[]})  [unwired: 1 in]
        }
        n362 = property on="Transcond Intensity" class="IntGraph (strict)"() -> ("Cursor.Cursor Plot"=w689:i32)  [unwired: 2 in, 2 out]
        n363 = local write "Conductance"(w699) -> ()
        n364 = property on="Horizontal Line Cut" class="XYGraph (strict)"() -> ("Cursor.Cursor Index"=w703:i32)  [unwired: 2 in, 2 out]
        "horizontal line cut\ncursor index" <- w703
        n365 = call <vilib>:"Add State(s) to Queue__jki_lib_state_machine.vi"("State(s) in (\"\")"=w721) -> ("States Out"=w720:string)  [unwired: 14 in]
        n366 = Index Array(array=w715, index=w689) -> (element=w706:cluster{"N1 (B field)":dbl[], dbl[]})
        n367 = property on="Vertical Line Cut" class="XYGraph (strict)"() -> ("Cursor.Cursor Index"=→"vertical line cut \ncursor index":i32)  [unwired: 2 in, 2 out]
        n368 = Build Array(w706) -> (→"Horizontal Line Cut":cluster{"N1 (B field)":dbl[], dbl[]}[])
        n369 = Bundle By Name(cluster=w682, "resample index"=w703) -> (w704:T14)
      }
      frame "Process: Export to igor" {
        n370 = local read "Blob File Path"() -> (w770:path)
        n371 = Strip Path(path=w770) -> (name=w775:string)  [unwired: 1 out]
        n372 = xnode "Match Regular Expression"("input string"=w775, "regular expression"=" -") -> ("before match"=w773:string)  [unwired: 4 in, 4 out]
        n373 = case shown="\"xy\"" "Enum" {
          tunnel: w773 -> [w912 w938 w956 w1036]
          tunnel: "export to igor path" -> [w906 w924 w949 w1023]
          tunnel: "xy graph X,Y,Z Scale Names" -> [_ _ w952 _]
          tunnel: "xy input ITX commands" -> [_ _ w958 _]
          tunnel: "intensity input ITX commands" -> [w918 w941 _ w1047]
          tunnel: "trans cond X,Y,Z Scale Names" -> [w899 w927 w953 _]
          tunnel: "cond int X,Y,Z Scale Names" -> [_ _ _ w1025]
          frame "Trans intensity", Default {
            # "#todo\nneed a place for these\ncommands\n(decipher commands)"
            n374 = local read "Transcond Intensity"() -> (w908:dbl[][])
            n375 = property on="Transcond Intensity" class="IntGraph (strict)"() -> ("ZScale.Minimum"=w917:dbl, "ZScale.Maximum"=w916:dbl)  [unwired: 2 in, 2 out]
            n376 = property on="Transcond Intensity" class="IntGraph (strict)"() -> ("XScale.Ofst&Mult"=w910:T19, "YScale.Ofst&Mult"=w909:T19)  [unwired: 2 in, 2 out]
            n377 = Number To Fractional String(number=w917) -> (F-format string=w922:string)  [unwired: 3 in]
            n378 = Number To Fractional String(number=w916) -> (F-format string=w920:string)  [unwired: 3 in]
            n379 = Array Size(array=w908) -> (size(s)=w915:i32[])
            n380 = Concatenate Strings(w912, "_trans" ("string")) -> (w905:string)
            n381 = Index Array(array=w915) -> (element #1=w914:i32, element #2=w913:i32)  [unwired: 2 in]
            n382 = call <userlib>:"Offset and Multiplier to Array.vi"("Size"=w914, "Offset and Multiplier"=w910) -> ("Array"=w903:dbl[])
            n383 = Concatenate Strings(w918, "\nModifyImage '#wave2D#' ctab= {", w922, ",", w920, ",YellowHot,0}") -> (w900:string)
            n384 = call <userlib>:"Offset and Multiplier to Array.vi"("Size"=w913, "Offset and Multiplier"=w909) -> ("Array"=w902:dbl[])
            n385 = Build Path(base path=w906, name or relative path=w905) -> (appended path=w901:path)
            n386 = Bundle By Name(cluster=T13 {"2D Array"=[], "X 1D Array"=[], "Y 1D Array"=[]} ("2D, X, Y (Cluster)"), "2D Array"=w908, "X 1D Array"=w903, "Y 1D Array"=w902) -> (w904:T13)
            n387 = flat-sequence {
              tunnel: w900 -> [_]
              frame #0 {
              }
            }
            n388 = call <userlib>:"LV to ITX 2D AutoPlot.vi"("X,Y,Z Labels"=w899, "2D, X, Y (Cluster)"=w904, "path"=w901) -> ()  [unwired: 7 in, 2 out]
          }
          frame "Flattened trans intensity" {
            # "#todo\nneed a place for these\ncommands\n(decipher commands)"
            n389 = property on="Flattened Trans" class="IntGraph (strict)"() -> ("ZScale.Minimum"=w940:dbl, "ZScale.Maximum"=w939:dbl)  [unwired: 2 in, 2 out]
            n390 = property on="Flattened Trans" class="IntGraph (strict)"() -> ("XScale.Ofst&Mult"=w925:T19, "YScale.Ofst&Mult"=w936:T19)  [unwired: 2 in, 2 out]
            n391 = local read "Flattened Trans"() -> (w931:dbl[][])
            n392 = Number To Fractional String(number=w940) -> (F-format string=w943:string)  [unwired: 3 in]
            n393 = Number To Fractional String(number=w939) -> (F-format string=w945:string)  [unwired: 3 in]
            n394 = Array Size(array=w931) -> (size(s)=w947:i32[])
            n395 = Concatenate Strings(w938, "_trans" ("string")) -> (w934:string)
            n396 = Index Array(array=w947) -> (element #1=w948:i32, element #2=w926:i32)  [unwired: 2 in]
            n397 = call <userlib>:"Offset and Multiplier to Array.vi"("Size"=w948, "Offset and Multiplier"=w925) -> ("Array"=w930:dbl[])
            n398 = Concatenate Strings(w941, "\nModifyImage '#wave2D#' ctab= {", w943, ",", w945, ",YellowHot,0}") -> (w932:string)
            n399 = call <userlib>:"Offset and Multiplier to Array.vi"("Size"=w926, "Offset and Multiplier"=w936) -> ("Array"=w929:dbl[])
            n400 = Build Path(base path=w924, name or relative path=w934) -> (appended path=w933:path)
            n401 = Bundle By Name(cluster=T13 {"2D Array"=[], "X 1D Array"=[], "Y 1D Array"=[]} ("2D, X, Y (Cluster)"), "2D Array"=w931, "X 1D Array"=w930, "Y 1D Array"=w929) -> (w928:T13)
            n402 = flat-sequence {
              tunnel: w932 -> [_]
              frame #0 {
              }
            }
            n403 = call <userlib>:"LV to ITX 2D AutoPlot.vi"("X,Y,Z Labels"=w927, "2D, X, Y (Cluster)"=w928, "path"=w933) -> ()  [unwired: 7 in, 2 out]
          }
          frame "xy" {
            # "#todo\nneed a place for these\ncommands"
            n404 = case shown="\"trans all\"" "xy graph data" {
              tunnel: [w967 w986 w1009 w1011] -> w959
              tunnel: [w972 w991 w998 w1018] -> w957
              tunnel: w956 -> [w964 w983 w1001 w1014]
              tunnel: [w962 w981 w1000 w1012] -> w950
              tunnel: w953 -> [_ w980 _ _]
              tunnel: [w961 w979 w997 w1010] -> w954
              tunnel: w952 -> [w961 _ w997 w1010]
              frame "cond all", Default {
                w969 = i16 0 ("precision (6)")
                w965 = "\n"
                w970 = " T\""
                n405 = local read "end B"() -> (w974:dbl)
                n406 = local read "start B"() -> (w973:dbl)
                n407 = local read "Conductance"() -> (w967:cluster{"N1 (B field)":dbl[], dbl[]}[])
                n408 = Concatenate Strings(w964, "") -> (w962:string)
                n409 = Number To Fractional String(number=w974, precision (6)=w969) -> (F-format string=w971:string)  [unwired: 2 in]
                n410 = Number To Fractional String(number=w973, precision (6)=w969) -> (F-format string=w976:string)  [unwired: 2 in]
                n411 = Concatenate Strings("\nTextBox/C/N=text0 \"\\\\f02B\\\\f00 = ", w976, w970, w965, "TextBox/C/N=text1 \"\\\\f02B\\\\f00 = ", w971, w970, w965, "SetAxis left 0,15", w965, "TextBox/C/N=text0/D=0.5\nTextBox/C/N=text1/D=0.5", w965) -> (w972:string)
              }
              frame "trans all" {
                w988 = i16 0 ("precision (6)")
                w984 = "\n"
                w989 = " T\""
                n412 = local read "end B"() -> (w993:dbl)
                n413 = local read "start B"() -> (w992:dbl)
                n414 = local read "Transconductance"() -> (w986:T4)
                n415 = Delete From Array(array=w980, length=1) -> (array with subset deleted=w979:string[])  [unwired: 1 in, 1 out]
                n416 = Concatenate Strings(w983, "_trans") -> (w981:string)
                n417 = Number To Fractional String(number=w993, precision (6)=w988) -> (F-format string=w990:string)  [unwired: 2 in]
                n418 = Number To Fractional String(number=w992, precision (6)=w988) -> (F-format string=w995:string)  [unwired: 2 in]
                n419 = Concatenate Strings("\nTextBox/C/N=text0 \"\\\\f02B\\\\f00 = ", w995, w989, w984, "TextBox/C/N=text1 \"\\\\f02B\\\\f00 = ", w990, w989, w984, "SetAxis left 0,15", w984, "TextBox/C/N=text0/D=0.5\nTextBox/C/N=text1/D=0.5", w984) -> (w991:string)
              }
              frame "horz cut" {
                w1002 = "\n"
                n420 = local read "Vsg (V)"() -> (w1007:dbl)
                n421 = Number To Fractional String(number=w1007, precision (6)=i16 1) -> (F-format string=w1006:string)  [unwired: 2 in]
                n422 = Concatenate Strings(w1001, "") -> (w1000:string)
                n423 = local read "Horizontal Line Cut"() -> (w1009:cluster{"N1 (B field)":dbl[], dbl[]}[])
                n424 = Concatenate Strings("\nTextBox/C/N=text0 \"\\\\f02V\\\\f00\\\\Bsg\\\\M = ", w1006, "mV", w1002, "TextBox/C/N=text0/D=0.5", w1002) -> (w998:string)
              }
              frame "vert cut" {
                w1015 = "\n"
                n425 = local read "B field (T)"() -> (w1022:dbl)
                n426 = local read "Vertical Line Cut"() -> (w1011:cluster{"N1 (B field)":dbl[], dbl[]}[])
                n427 = Concatenate Strings(w1014, "") -> (w1012:string)
                n428 = Number To Fractional String(number=w1022, precision (6)=i16 1) -> (F-format string=w1020:string)  [unwired: 2 in]
                n429 = Concatenate Strings("\nTextBox/C/N=text0 \"\\\\f02B\\\\f00 = ", w1020, " T\"", w1015, "TextBox/C/N=text0/D=0.5", w1015) -> (w1018:string)
              }
            }
            n430 = Build Path(base path=w949, name or relative path=w950) -> (appended path=w951:path)
            n431 = Concatenate Strings(w958, w957) -> (w955:string)
            n432 = flat-sequence {
              tunnel: w955 -> [_]
              frame #0 {
              }
            }
            n433 = call <userlib>:"LV to ITX XY AutoPlot.vi"("X,Y Labels"=w954, "XY-Data []"=w959, "path"=w951) -> ()  [unwired: 7 in, 2 out]
          }
          frame "Cond intensity" {
            # "#todo\n?"
            # "#todo\nneed a place for these\ncommands\n(decipher commands)"
            n434 = property on="Cond intensity" class="IntGraph (strict)"() -> ("ZScale.Minimum"=w1045:dbl, "ZScale.Maximum"=w1042:dbl)  [unwired: 2 in, 2 out]
            n435 = local read "Cond intensity"() -> (w1030:dbl[][])
            n436 = property on="Cond intensity" class="IntGraph (strict)"() -> ("XScale.Ofst&Mult"=w1031:T19, "YScale.Ofst&Mult"=w1032:T19)  [unwired: 2 in, 2 out]
            n437 = Concatenate Strings("_cond" ("string"), w1036) -> (w1027:string)
            n438 = Number To Fractional String(number=w1045) -> (F-format string=w1044:string)  [unwired: 3 in]
            n439 = Array Size(array=w1030) -> (size(s)=w1040:i32[])
            n440 = Index Array(array=w1040) -> (element #1=w1039:i32, element #2=w1038:i32)  [unwired: 2 in]
            n441 = Number To Fractional String(number=w1042) -> (F-format string=w1041:string)  [unwired: 3 in]
            n442 = call <userlib>:"Offset and Multiplier to Array.vi"("Size"=w1039, "Offset and Multiplier"=w1031) -> ("Array"=w1034:dbl[])
            n443 = call <userlib>:"Offset and Multiplier to Array.vi"("Size"=w1038, "Offset and Multiplier"=w1032) -> ("Array"=w1033:dbl[])
            n444 = Concatenate Strings(w1047, "\nModifyImage '#wave2D#' ctab= {", w1044, ",", w1041, ",YellowHot,0}") -> (w1028:string)
            n445 = Bundle By Name(cluster=T13 {"2D Array"=[], "X 1D Array"=[], "Y 1D Array"=[]} ("2D, X, Y (Cluster)"), "2D Array"=w1030, "X 1D Array"=w1034, "Y 1D Array"=w1033) -> (w1029:T13)
            n446 = Build Path(base path=w1023, name or relative path=w1027) -> (appended path=w1026:path)
            n447 = flat-sequence {
              tunnel: w1028 -> [_]
              frame #0 {
              }
            }
            n448 = call <userlib>:"LV to ITX 2D AutoPlot.vi"("X,Y,Z Labels"=w1025, "2D, X, Y (Cluster)"=w1029, "path"=w1026) -> ()  [unwired: 7 in, 2 out]
          }
        }
        n449 = call <vilib>:"Add State(s) to Queue__jki_lib_state_machine.vi"("State(s) in (\"\")"=w783) -> ("States Out"=w782:string)  [unwired: 14 in]
      }
    }
  }
